vi "运维调试_采配水V3.vi"() -> ()   [LabVIEW 2016, in "PLC.lvlib"]
uses:
  PLC.lvlib
  <vilib>/Plasmionique/MB Master/MB_Master/MB_Master.lvclass
  <vilib>/Utility/miscctls.llb/LVPointTypeDef.ctl
  <vilib>/Plasmionique/MB Master/MB_Master_Serial/MB_Master_Serial.lvclass
  C:/Program Files (x86)/National Instruments/LabVIEW 2016/vi.lib/Plasmionique/MB Master/MB_Master/MB_Master.lvclass
  <vilib>/Instr/_visa.llb/VISA Configure Serial Port (Instr).vi
  <vilib>/Plasmionique/MB Master/MB Master.lvlib
panel:
  out "Registers":u16[](array[numeric])
  out "R124":i16 caption="加标回收配水时间"
  out "R44":i16
  in  "V14":bool
  in  "更新程序":bool
  out "R122":i16 caption="二级自来水清洗时间"
  out "R121":i16 caption="一级自来水清洗时间"
  out "R120":i16 caption="过滤自来水清洗时间"
  out "清洗次数":u16
  out "当前启动泵号":u16(ring) items=["1号泵", "2号泵"]
  out "R116":i16 caption="储水时间"
  in  "R113":u16(ring) caption="水箱储水水体" items=["自来水", "水样"]
  out "R112":i16 caption="二级水样池进样超时"
  in  "R111":u16(ring) caption="采配水型号" items=["常规版本", "高配版本"]
  out "数值 19":dbl
  out "数值 18":dbl
  out "数值 17":dbl
  out "数值 16":dbl
  out "数值 15":dbl
  out "数值 14":dbl
  out "数值 13":dbl
  out "数值 12":dbl
  out "数值 11":dbl
  out "数值 10":dbl
  out "数值 9":dbl
  out "数值 8":dbl
  out "数值 7":dbl
  out "数值 6":dbl
  out "数值 5":dbl
  out "数值 4":dbl
  out "数值 3":dbl
  out "数值 2":dbl
  out "数值":dbl
  in  "R118":u16(ring) caption="是否启用质控" items=["不启用质控", "启用质控"]
  out "压力传感器":dbl format="%#.2f"
  out "R110":i16 caption="过滤装置排液时间"
  in  "M4":bool
  in  "M3":bool
  in  "V13":bool
  in  "V12":bool
  in  "V1-R":bool
  in  "V1-G":bool
  in  "V11":bool
  in  "V10":bool
  in  "V9":bool
  in  "V8":bool
  in  "V7-R":bool
  in  "V7-G":bool
  out "X2":bool caption="X1"
  out "采配水版本号":string
  out "R117":i16 caption="清洗频次设定"
  out "通讯故障":bool
  in  "R100":u16(ring) caption="采水泵工作模式" items=["泵1单泵单管路", "泵2单泵单管路", "潜水泵双泵双管路", "自吸泵双泵双管路"]
  out "X11":bool caption="自来水检测_WA"
  out "X10":bool caption="废液报警_WLA"
  out "X9":bool caption="泵2过载报警_KM2"
  out "X8":bool caption="泵1过载报警_KM1"
  out "X7":bool caption="断电检测_DD"
  out "X6":bool caption="门禁开关_MJ"
  out "X5":bool caption="烟雾检测_YW"
  out "X4":bool caption="浸水检测_SJ"
  out "X3":bool caption="水流开关_JY"
  out "X1":bool
  out "X0":bool caption="采样池液位开关_YE1"
  out "R109":i16 caption="外部反冲洗时间"
  out "集成报警信息":string
  out "R108":i16 caption="进样超时时间"
  out "R107":i16 caption="进气时间"
  out "R106":i16 caption="排液时间"
  out "R105":i16 caption="常规模式配水时间"
  out "R104":i16 caption="过滤次数"
  out "R103":i16 caption="过滤配水时间"
  out "R102":i16 caption="一级沉淀时间"
  out "R101":i16 caption="管路润洗时间"
  out "R2":i16
  out "R1":i16
  out "多列列表框":i32(listbox)
  in  "V6":bool
  in  "V5":bool
  in  "V4":bool
  in  "V3":bool
  in  "V2":bool
  in  "M2":bool
  in  "M1":bool
  in  "返回":bool
  in  "参数设置":bool
  in  "单步启动":bool
  in  "启动":bool
  in  "停止":bool
  # "流程计时："
  # "s"
  # "压力传感器："
  # "MPa"
  # "二级液位开关低_Y2FD"
  # "二级液位开关高_YF2H"
  # "S"
  # "S"
  # "S"
  # "S"
  # "S"
  # "S"
  # "次"
  # "S"
  # "S"
  # "S"
  # "S"
  # "S"
  # "S"
  # "单步计时："
  # "s"
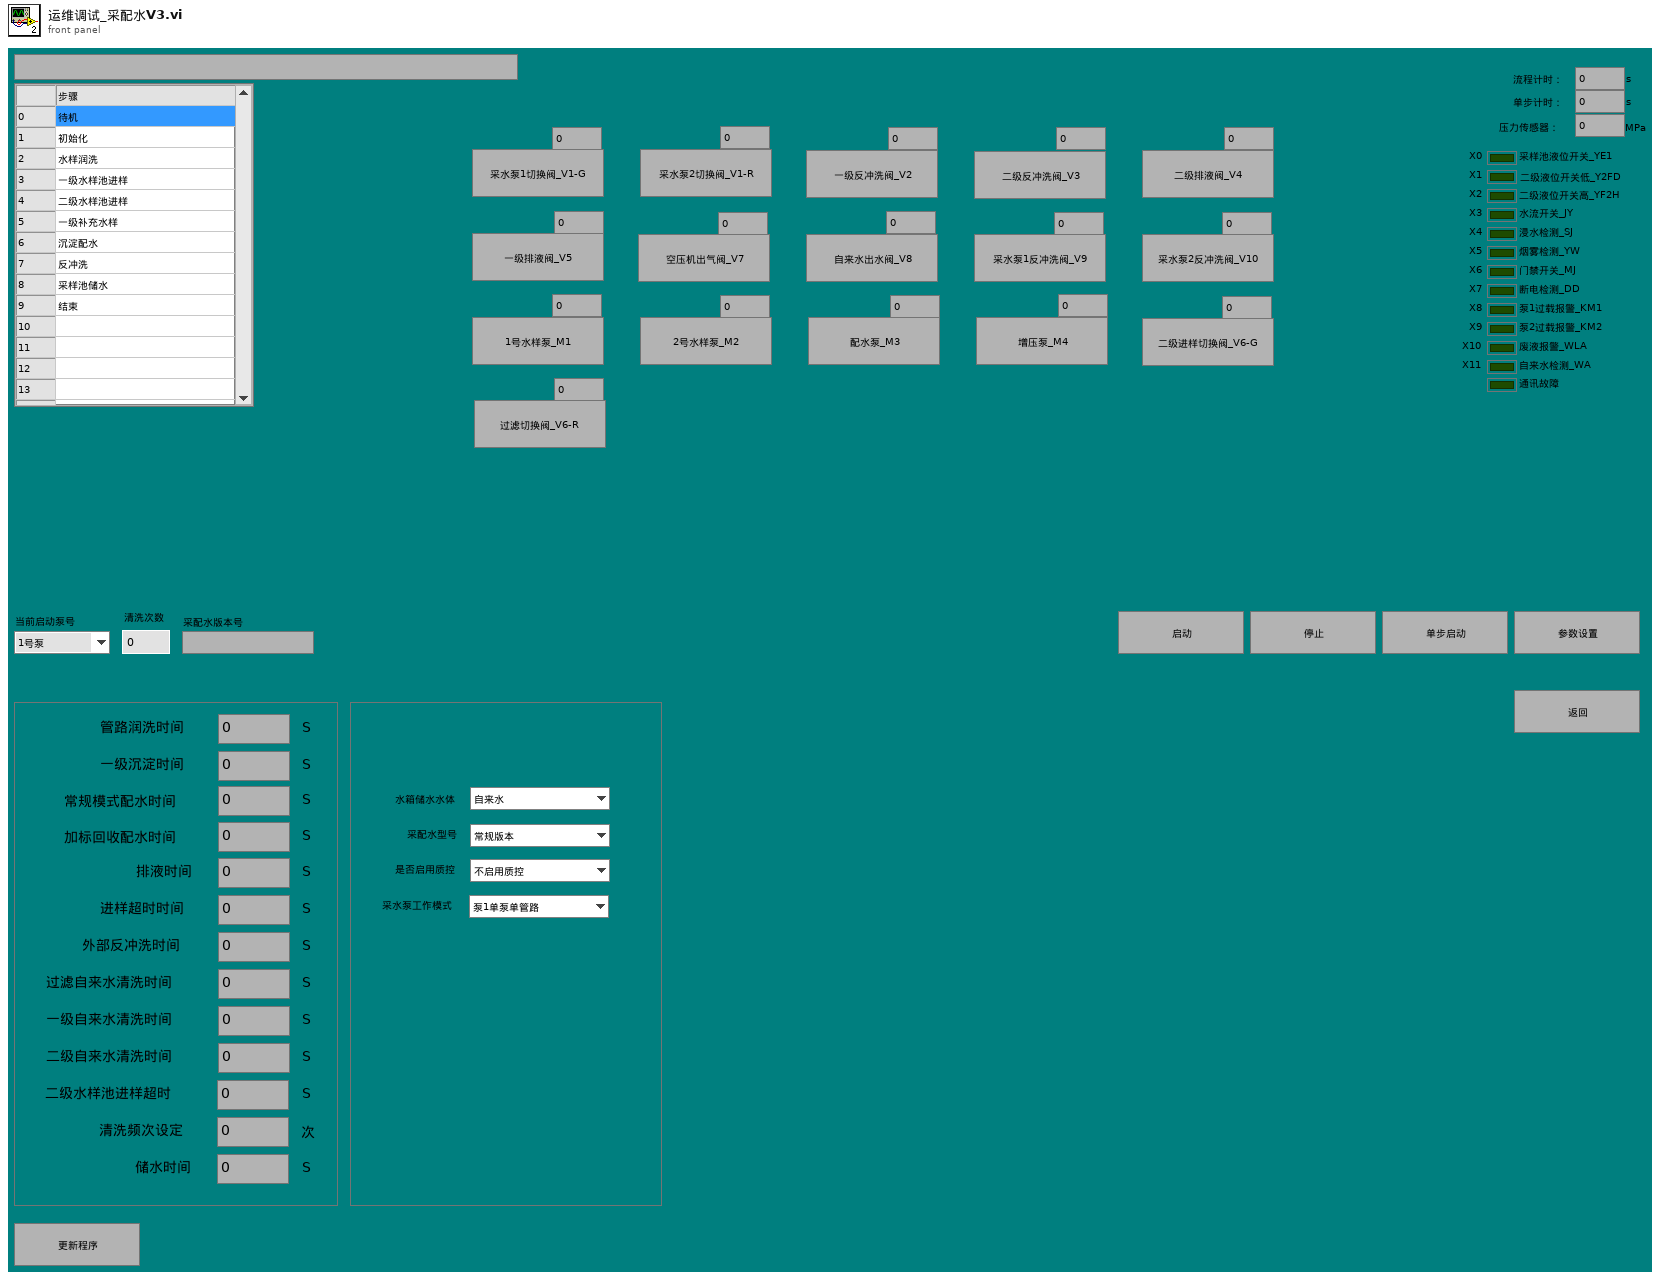
[diagram p1: front panel]
types:
  T1 = cluster{"测试模式":enum16{"水样测试", "平行样测试", "集成干预测试", "加标回收"}, "参数启用":cluster{"氨氮":bool, "总磷":bool, "总氮":bool, "多参数":bool, "CODMn":bool, "CODcr":bool, "超标留样":bool}}
  T2 = typedef "LVPointTypeDef.ctl" = cluster{"Horizontal":i16, "Vertical":i16}
  T3 = cluster{"命令":string, "数据":cluster{"starting address":u16, "holding register value":u16}}
  T4 = cluster{"命令":string, cluster{"starting address":u16, "holding register value":u16}}
  T5 = cluster{"命令":string, "数据":cluster{"starting address":u16, "holding register values":u16[]}}
  T6 = cluster{"命令":string, "data":cluster{"starting address":u16, "coil values":bool[]}}
  T7 = cluster{"参数启用":cluster{"氨氮":bool, "总磷总氮":bool, "总氮":bool, "多参数":bool, "CODMn":bool, "CODcr":bool, "超标留样":bool}}
  T8 = cluster{"氨氮":bool, "总磷总氮":bool, "总氮":bool, "多参数":bool, "CODMn":bool, "CODcr":bool, "超标留样":bool}
  T9 = cluster{"测试模式":enum16{"水样测试", "平行样测试", "集成干预测试", "加标回收"}, "参数启用":cluster{"氨氮":bool, "总磷总氮":bool, "总氮":bool, "多参数":bool, "CODMn":bool, "CODcr":bool, "超标留样":bool}}
  T10 = cluster{"R0":i16, "R1":i16, "R2":i16, "R3":i16, "R4":i16, "R5":i16, "R6":i16, "R7":i16, "R8":i16, "R9":i16, "R10":i16, "R11":i16, "R12":i16, "R13":i16, "R14":i16, "R15":i16, "R16":i16, "R17":i16, "R18":i16, "R19":i16, "R20":i16, "R21":i16, "R22":i16, "R23":i16, "R24":i16, "R25":i16, "R26":i16, "R27":i16, "R28":i16, "R29":i16, "R30":i16, "R31":i16, "R32":i16, "R33":i16, "R34":i16, "R35":i16, "R36":i16, "R37":i16, "R38":i16, "R39":i16, "R40":i16, "R41":i16, "R42":i16, "R43":i16, "R44":i16, "R45":i16, "R46":i16, "R47":i16, "R48":i16, "R49":i16, "R50":i16, "R51":i16, "R52":i16, "R53":i16, "R54":i16, "R55":i16, "R56":i16, "R57":i16, "R58":i16, "R59":i16, "R60":i16, "R61":i16, "R62":i16, "R63":i16, "R64":i16, "R65":i16, "R66":i16, "R67":i16, "R68":i16, "R69":i16, "R70":i16, "R71":i16, "R72":i16, "R73":i16, "R74":i16, "R75":i16, "R76":i16, "R77":i16, "R78":i16, "R79":i16}
  T11 = cluster{"seconds since 1Jan1904":timestamp, "table输入":string, string, "table输入":string}
  T12 = cluster{"baud rate (bps)":u32, "stop bits":u16, "parity":u16, "flow control":u16, "timeout":u32, "retries":i32}
  T13 = cluster{"starting address":u16, "holding register values":u16[]}
  T14 = cluster{"starting address":u16, "holding register value":u16}
  T15 = cluster{"starting address":u16, "coil values":bool[]}
  T16 = cluster{"Registers[0]":u16, "Registers[1]":u16, "Registers[2]":u16, "Registers[3]":u16, "Registers[4]":u16, "Registers[5]":u16, "Registers[6]":u16, "Registers[7]":u16, "Registers[8]":u16, "Registers[9]":u16, "Registers[10]":u16, "Registers[11]":u16, "Registers[12]":u16, "Registers[13]":u16, "Registers[14]":u16, "Registers[15]":u16, "Registers[16]":u16, "Registers[17]":u16, "Registers[18]":u16, "Registers[19]":u16, "Registers[20]":u16, "Registers[21]":u16, "Registers[22]":u16, "Registers[23]":u16, "Registers[24]":u16, "Registers[25]":u16, "Registers[26]":u16, "Registers[27]":u16, "Registers[28]":u16, "Registers[29]":u16, "Registers[30]":u16, "Registers[31]":u16, "Registers[32]":u16, "Registers[33]":u16, "Registers[34]":u16, "Registers[35]":u16, "Registers[36]":u16, "Registers[37]":u16, "Registers[38]":u16, "Registers[39]":u16, "Registers[40]":u16, "Registers[41]":u16, "Registers[42]":u16, "Registers[43]":u16, "Registers[44]":u16, "Registers[45]":u16, "Registers[46]":u16, "Registers[47]":u16, "Registers[48]":u16, "Registers[49]":u16, "Registers[50]":u16, "Registers[51]":u16, "Registers[52]":u16, "Registers[53]":u16, "Registers[54]":u16, "Registers[55]":u16, "Registers[56]":u16, "Registers[57]":u16, "Registers[58]":u16, "Registers[59]":u16, "Registers[60]":u16, "Registers[61]":u16, "Registers[62]":u16, "Registers[63]":u16, "Registers[64]":u16, "Registers[65]":u16, "Registers[66]":u16, "Registers[67]":u16, "Registers[68]":u16, "Registers[69]":u16, "Registers[70]":u16, "Registers[71]":u16, "Registers[72]":u16, "Registers[73]":u16, "Registers[74]":u16, "Registers[75]":u16, "Registers[76]":u16, "Registers[77]":u16, "Registers[78]":u16, "Registers[79]":u16}
  T17 = cluster{"Registers[0]":u16, "Registers[1]":u16, "Registers[2]":u16, "Registers[3]":u16, "Registers[4]":u16, "Registers[5]":u16}
  T18 = cluster{"Registers[0]":u16, "Registers[1]":u16, "Registers[2]":u16, "Registers[3]":u16, "Registers[4]":u16, "Registers[5]":u16, "Registers[6]":u16, "Registers[7]":u16, "Registers[8]":u16, "Registers[9]":u16, "Registers[10]":u16, "Registers[11]":u16, "Registers[12]":u16, "Registers[13]":u16, "Registers[14]":u16, "Registers[15]":u16, "Registers[16]":u16, "Registers[17]":u16, "Registers[18]":u16, "Registers[19]":u16, "Registers[20]":u16, "Registers[21]":u16, "Registers[22]":u16, "Registers[23]":u16, "Registers[24]":u16, "Registers[25]":u16, "Registers[26]":u16, "Registers[27]":u16, "Registers[28]":u16, "Registers[29]":u16, "Registers[30]":u16, "Registers[31]":u16, "Registers[32]":u16, "Registers[33]":u16}
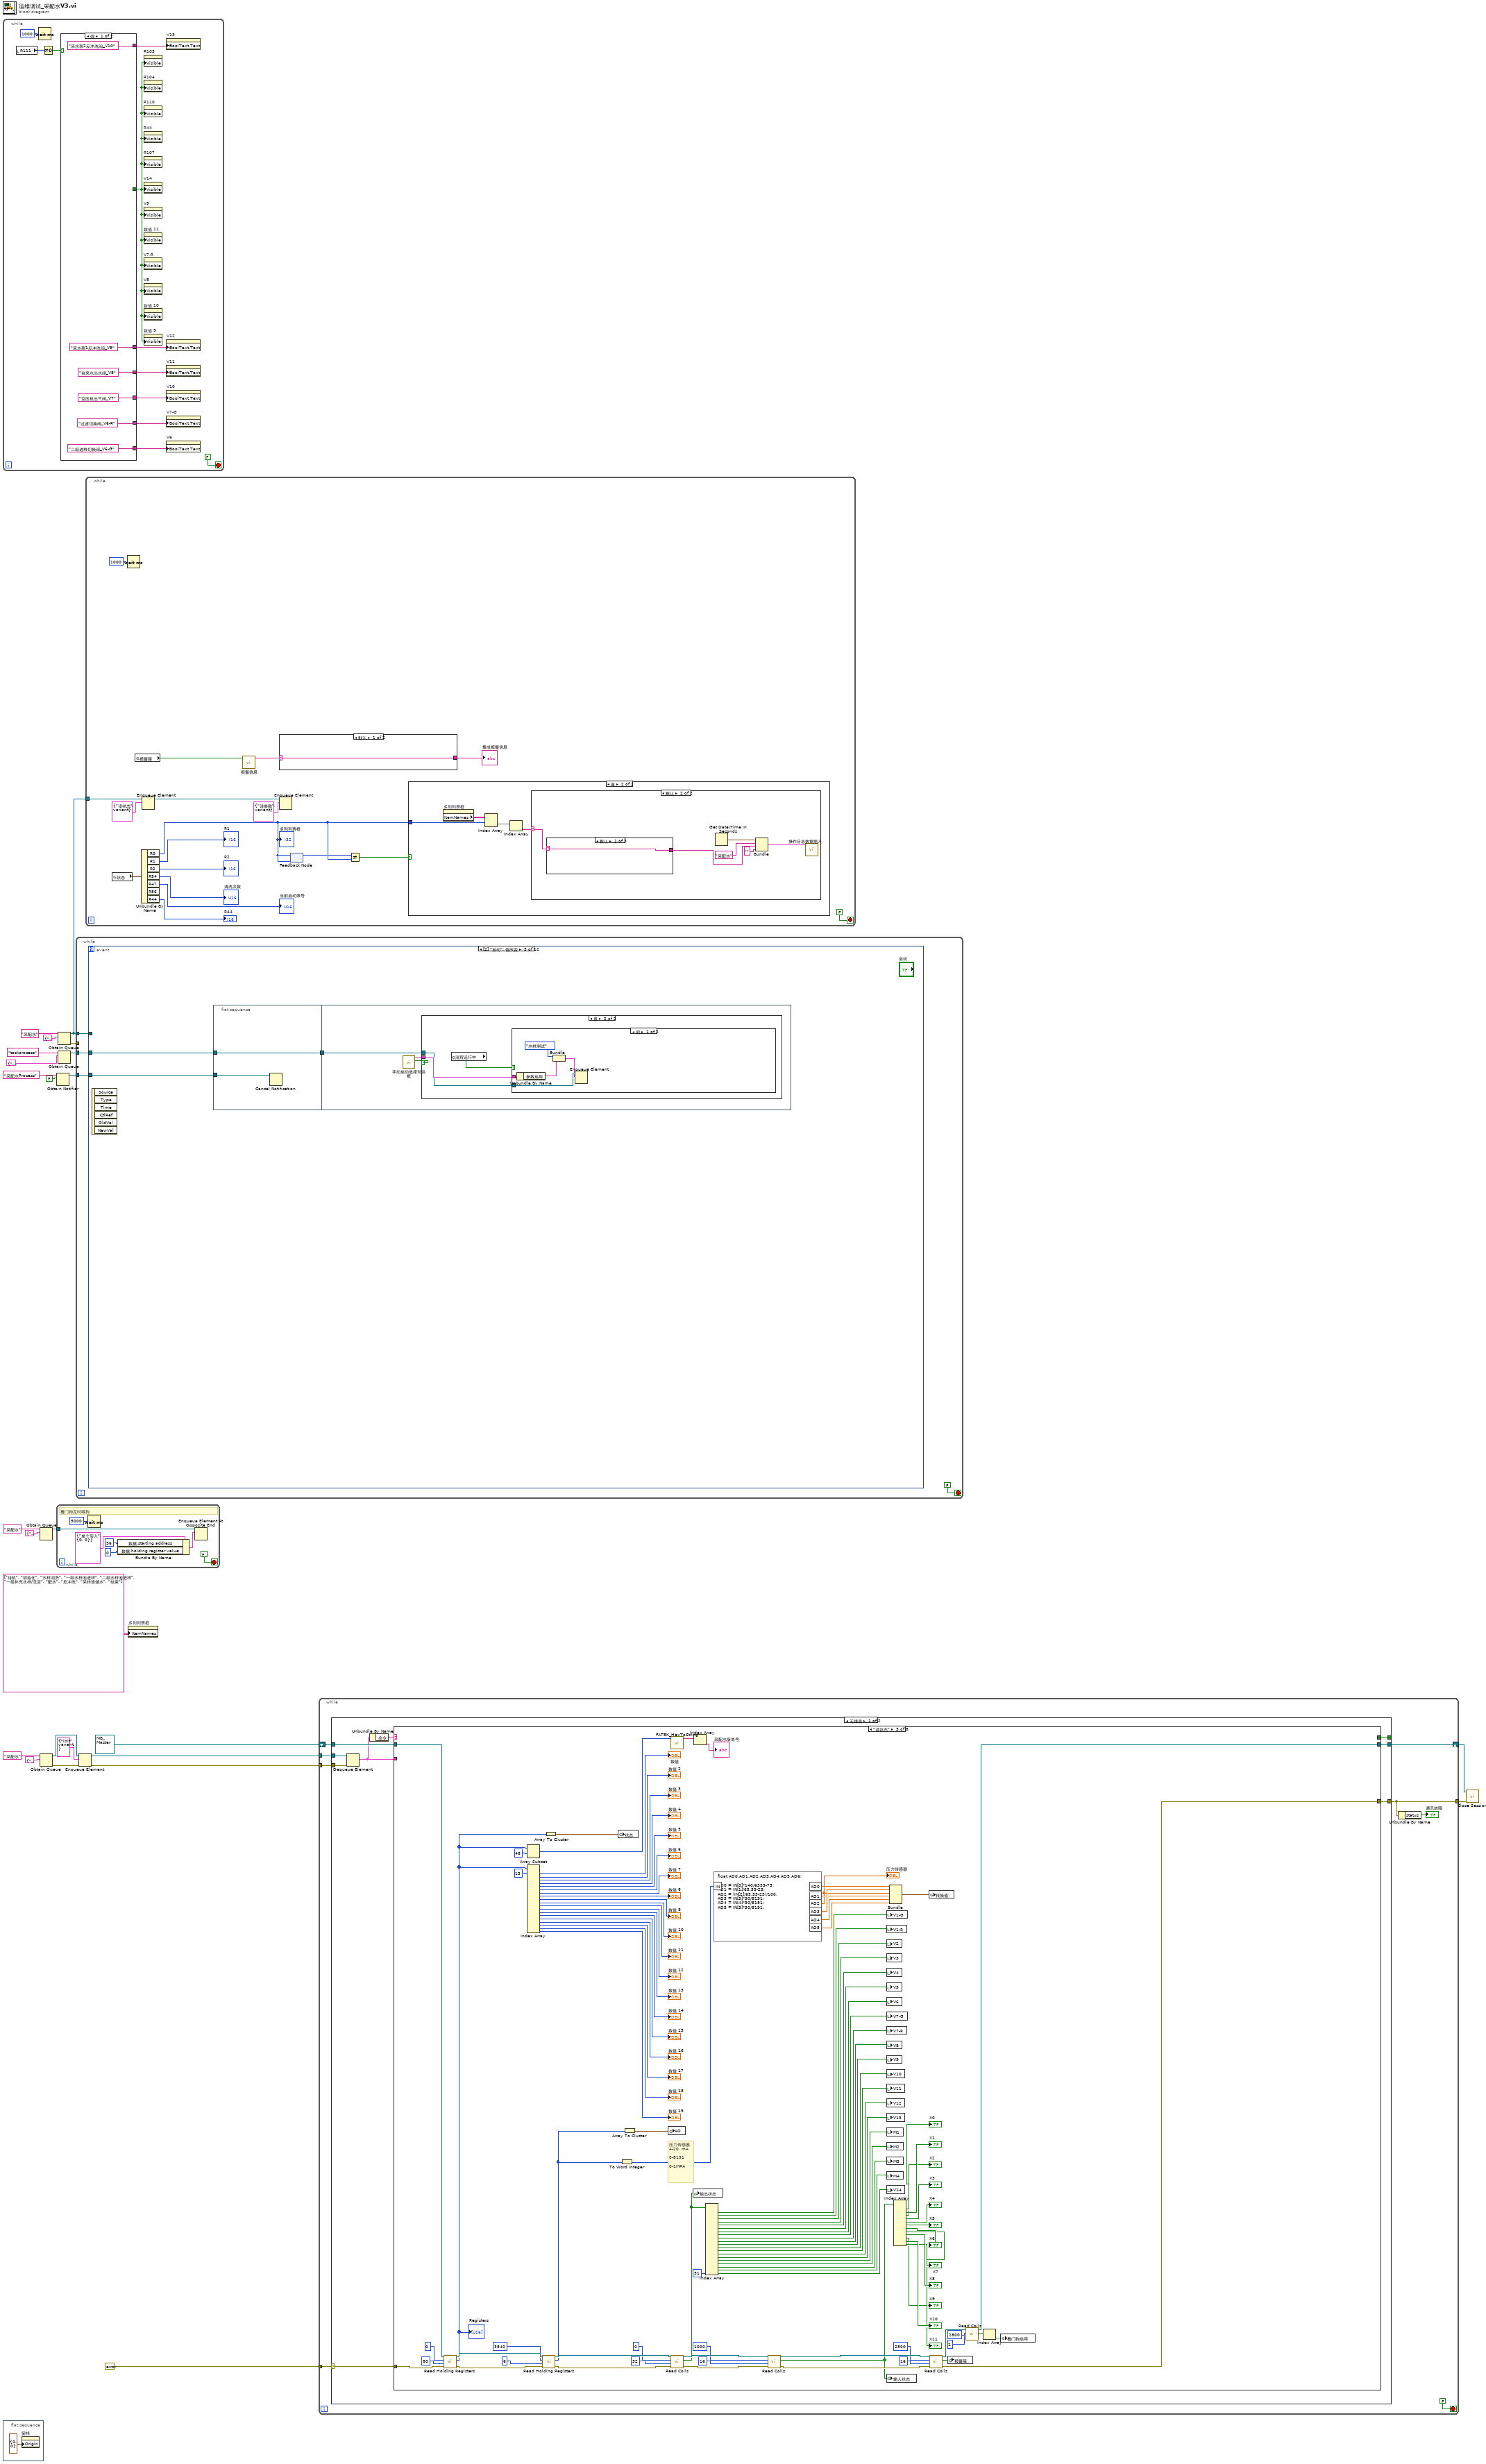
[diagram p0: block diagram]
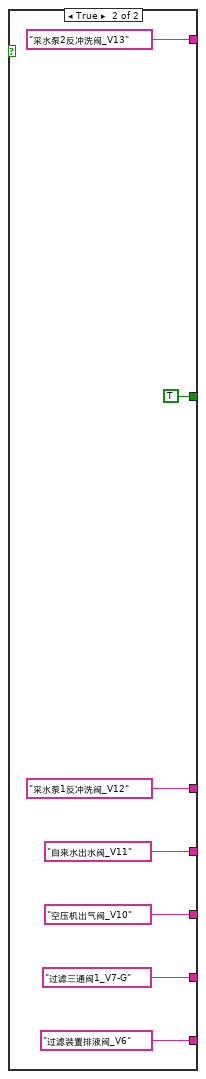
[diagram p2: hidden frame]
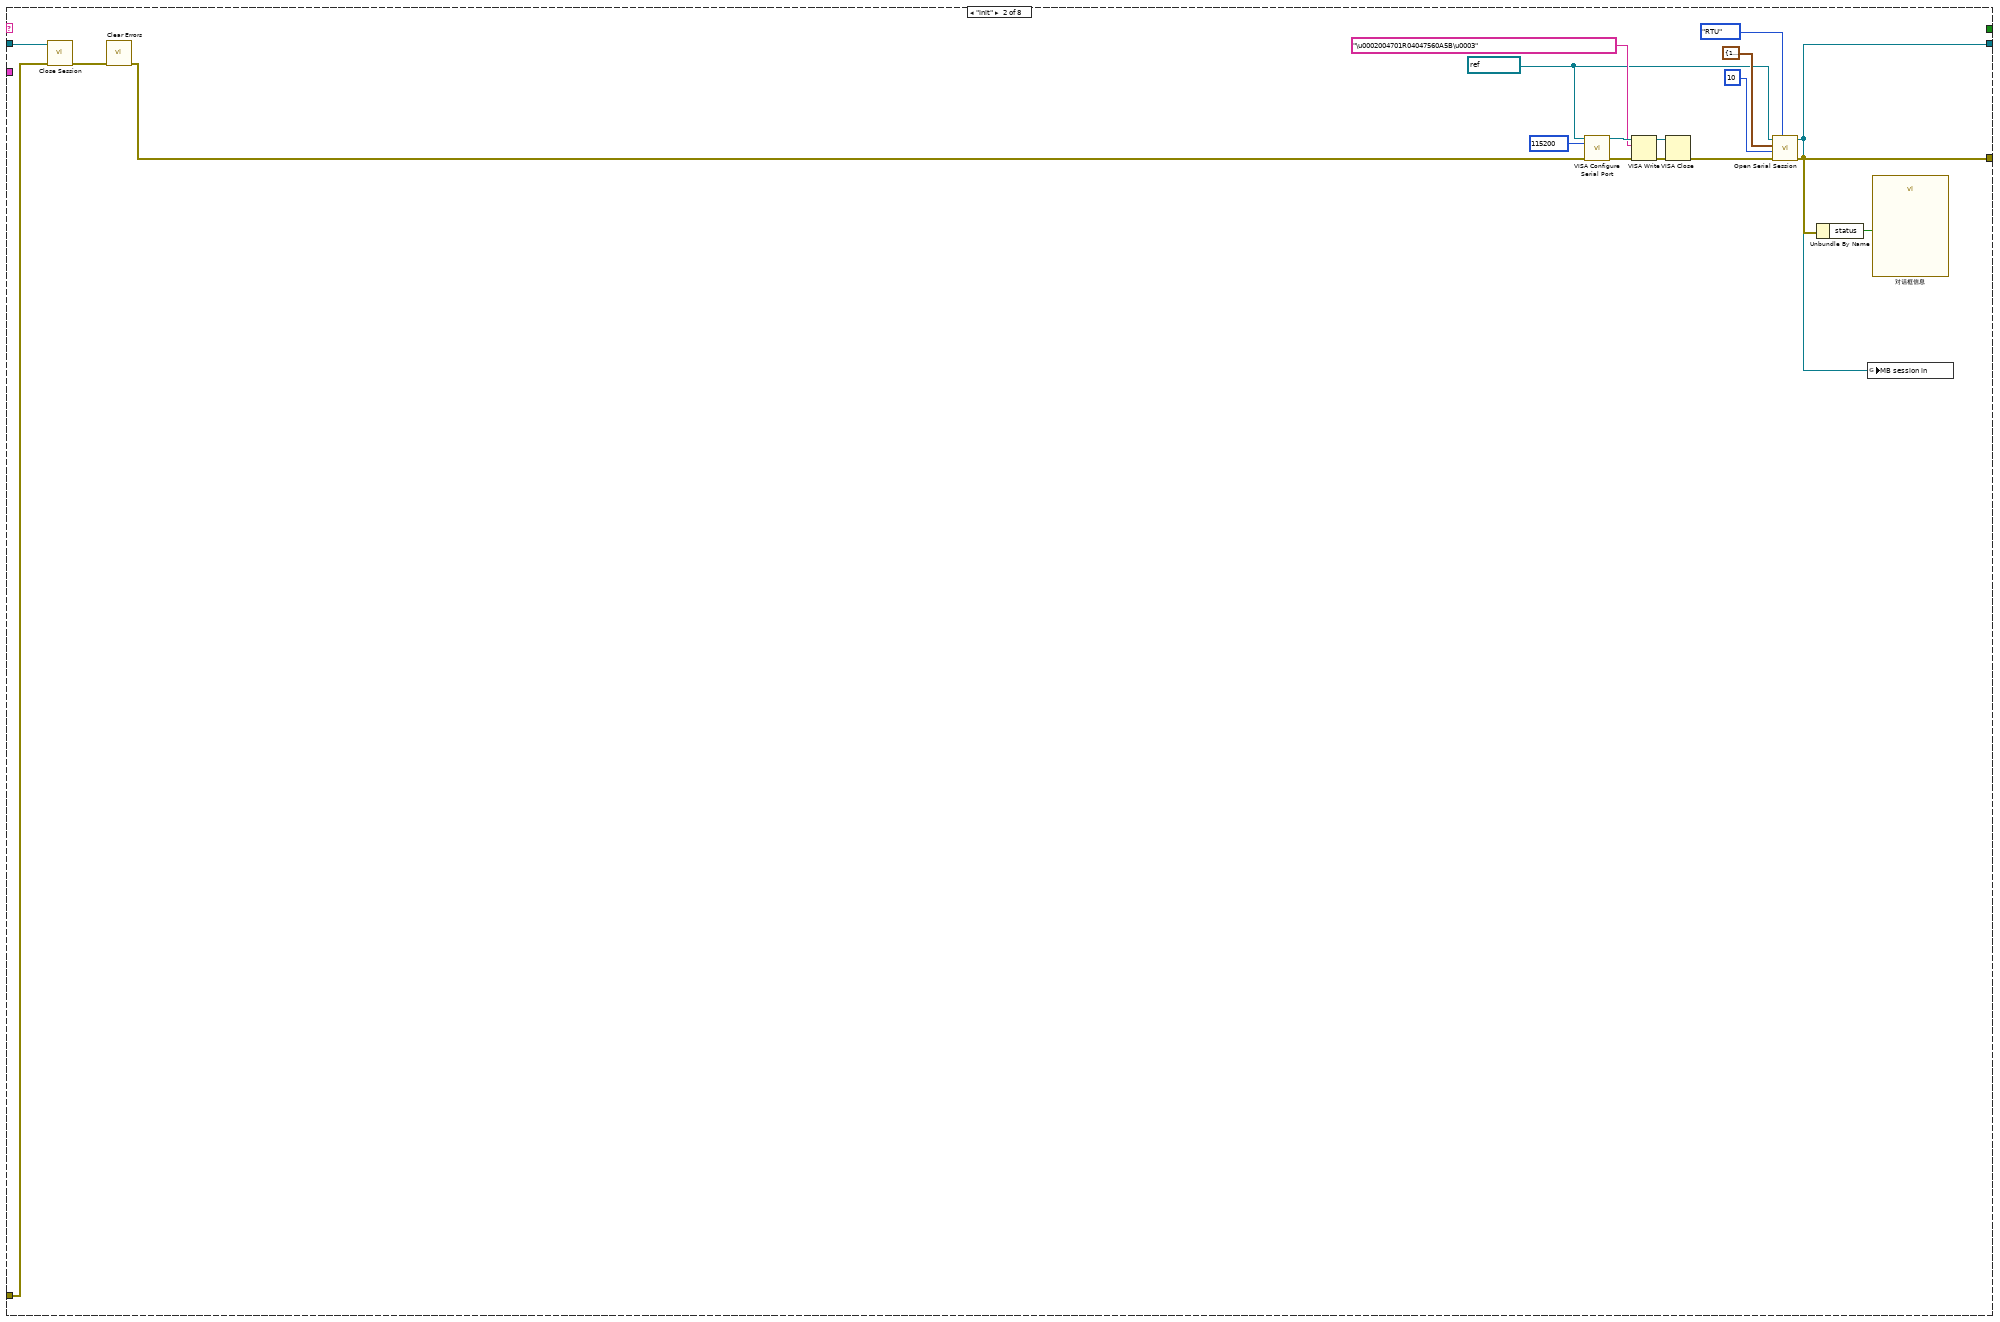
[diagram p4: hidden frame]
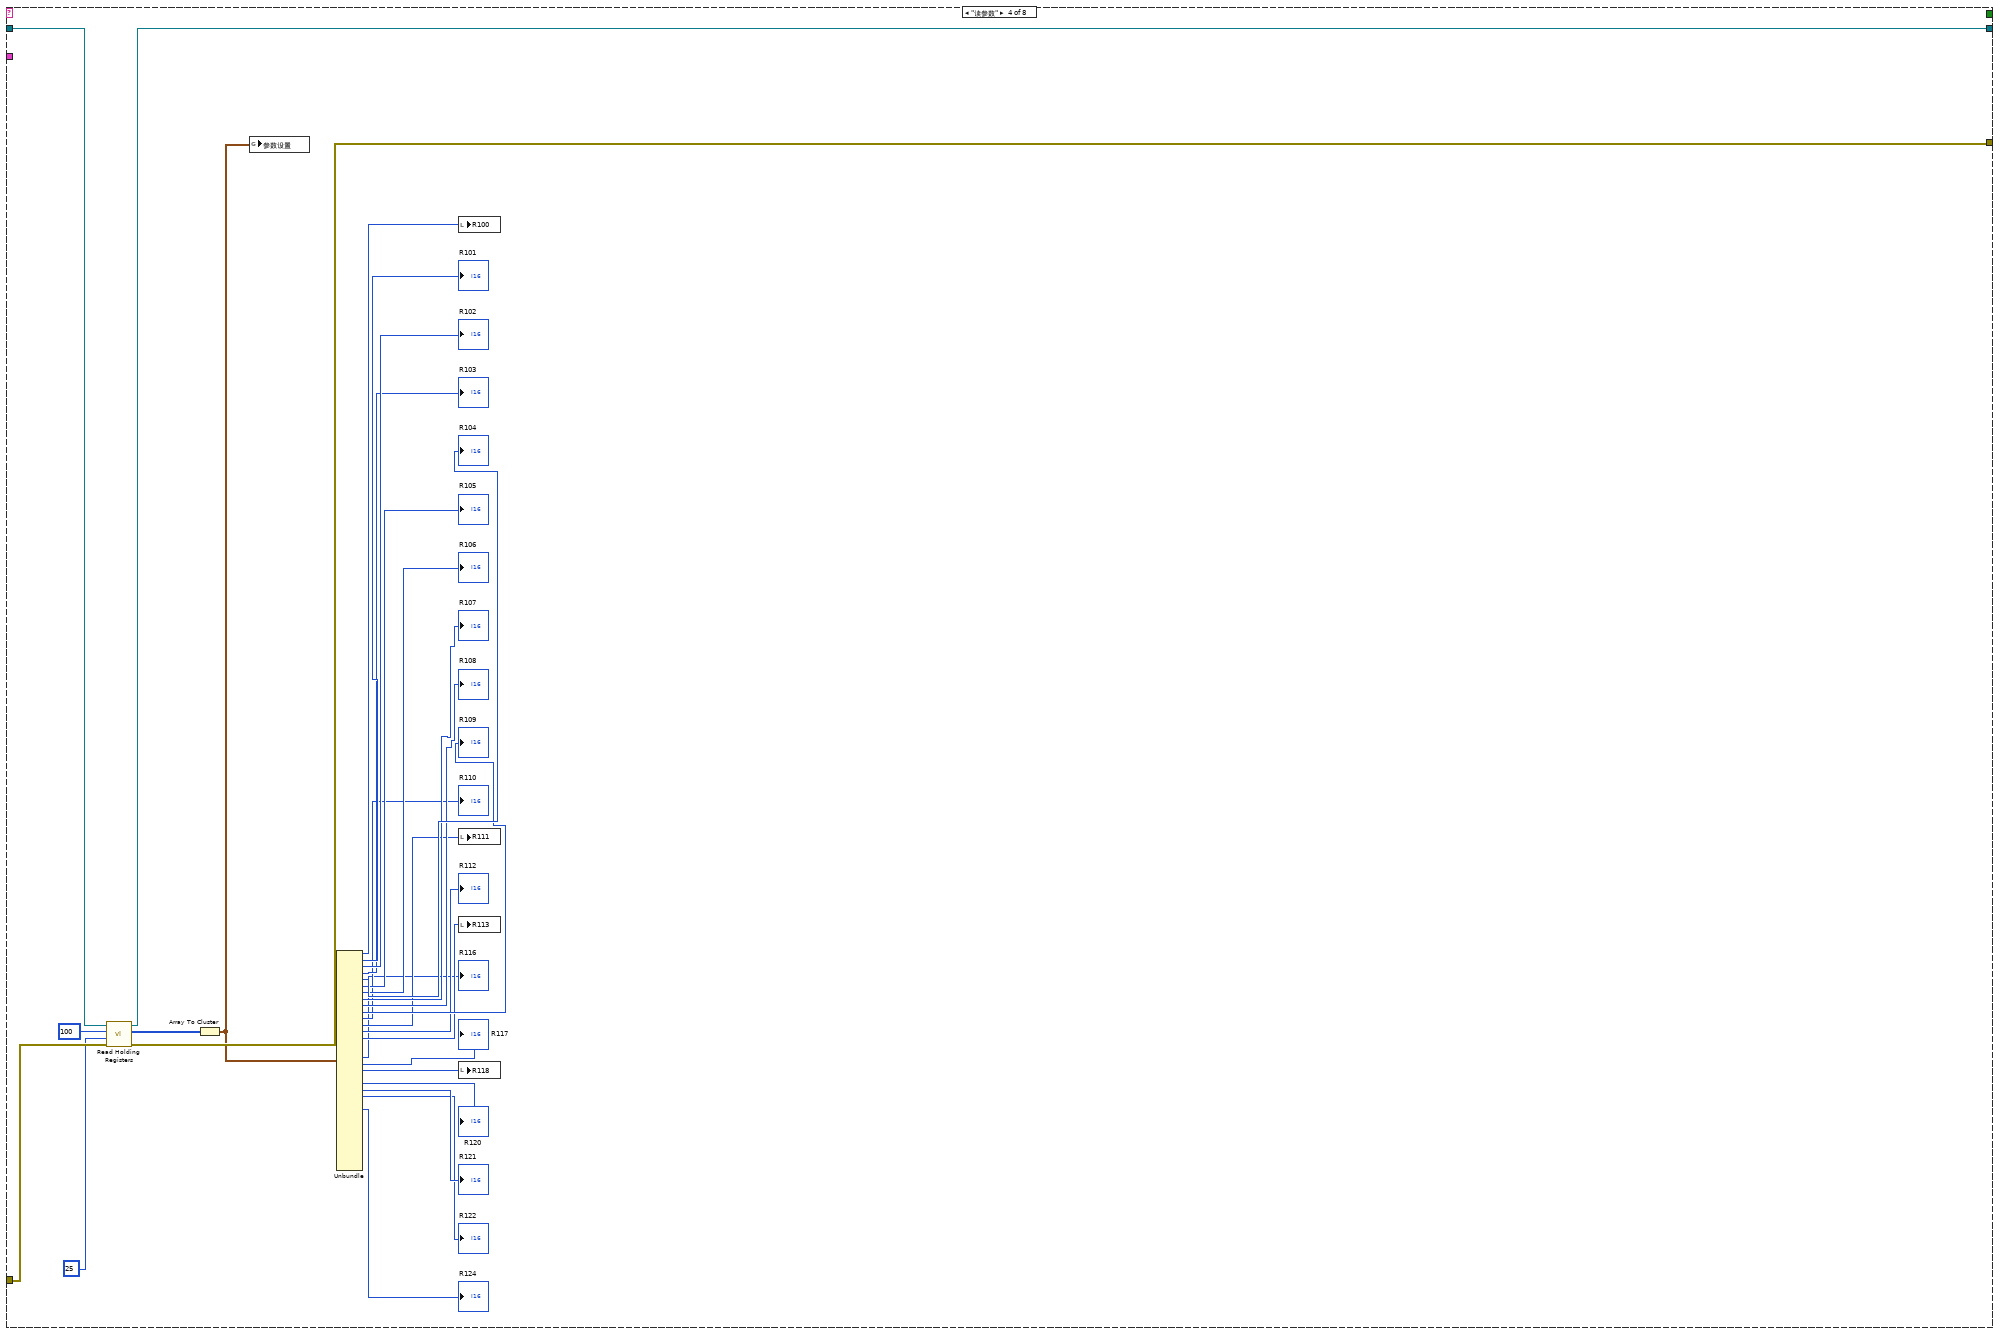
[diagram p5: hidden frame]
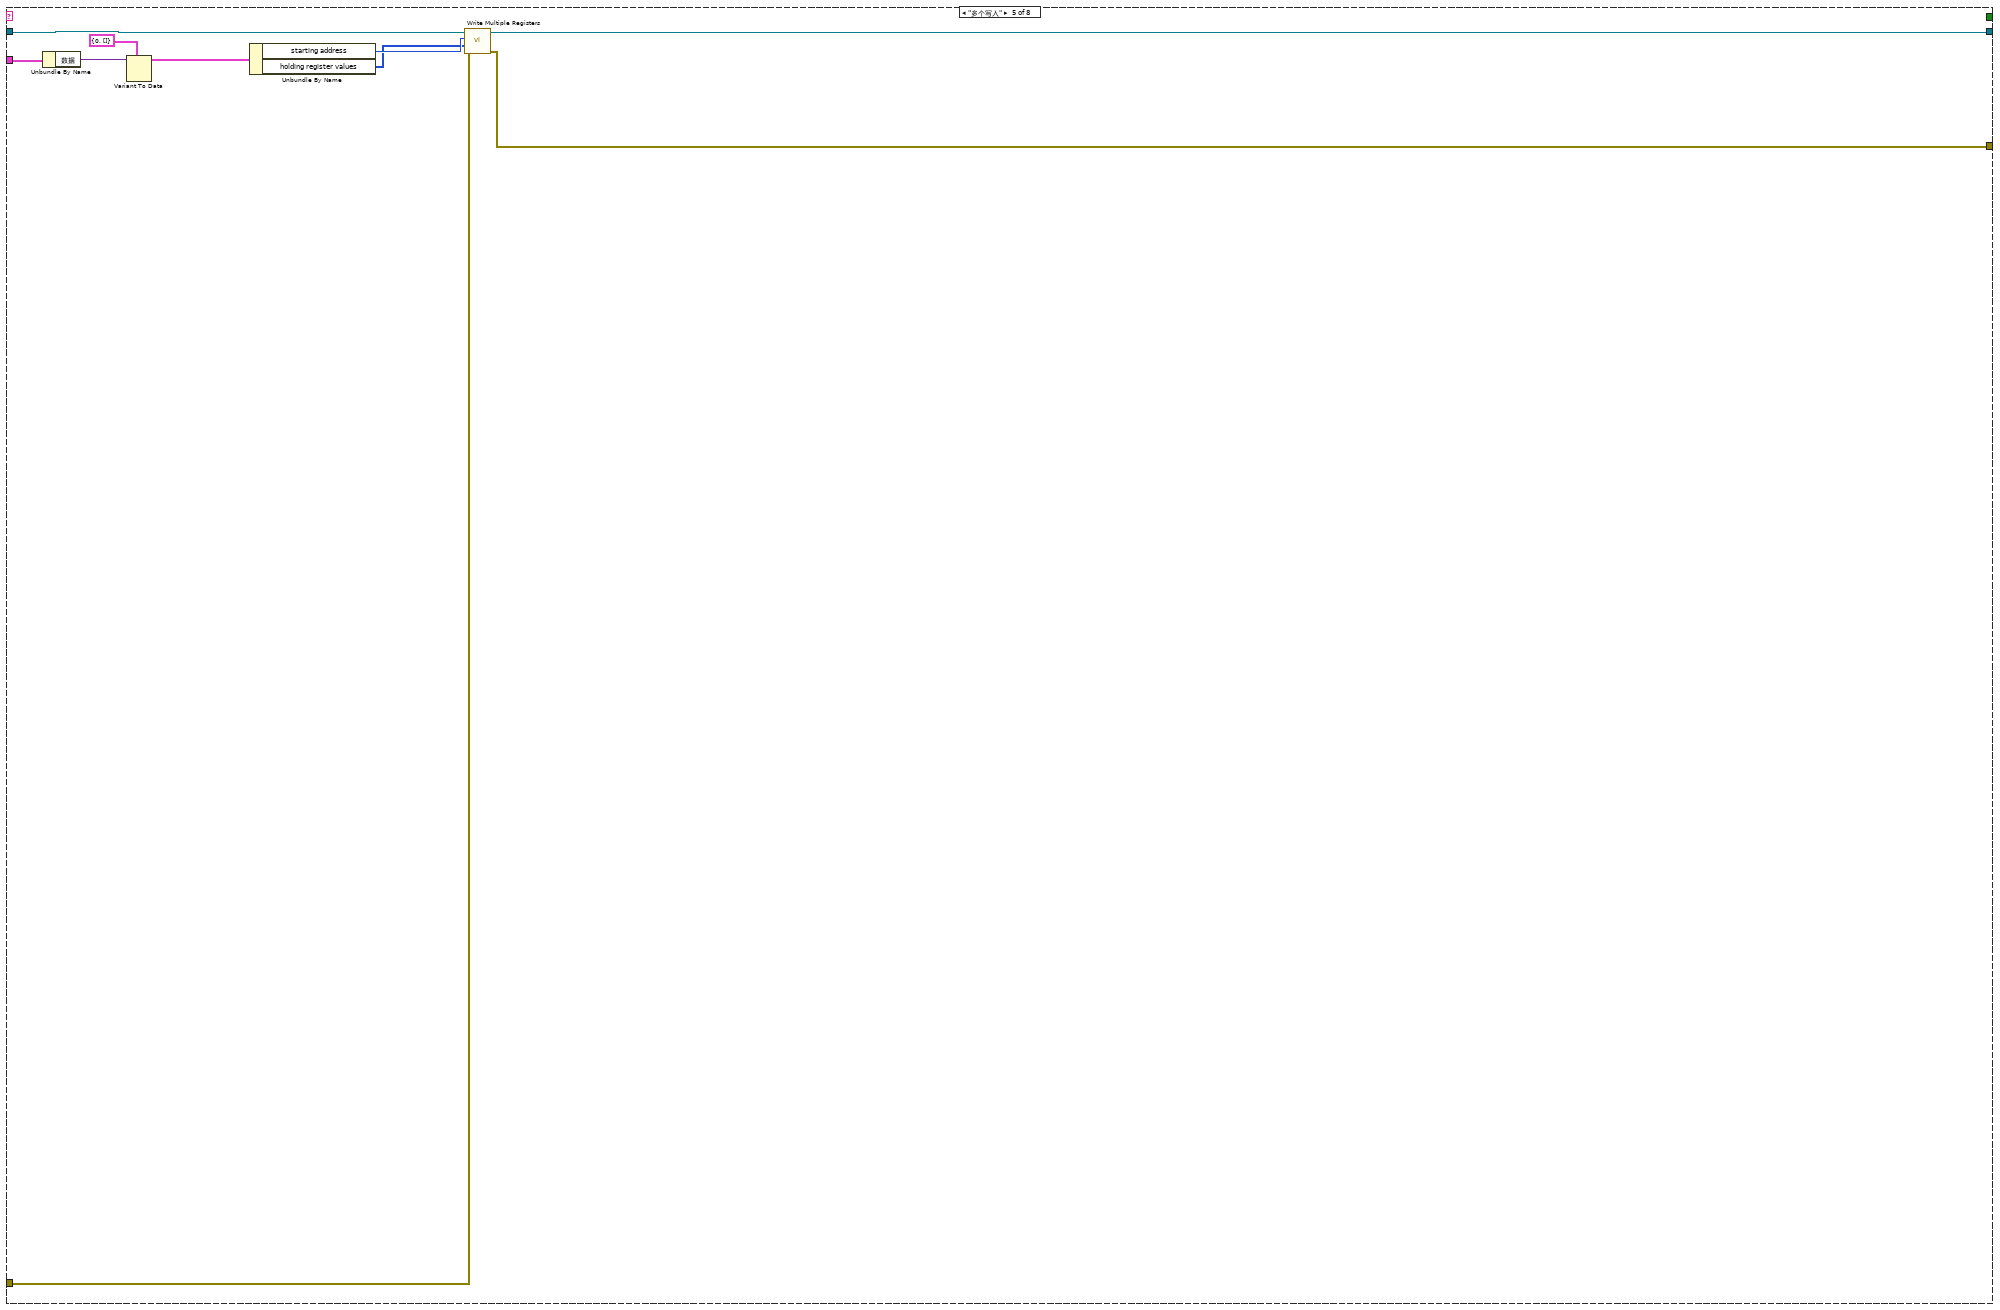
[diagram p6: hidden frame]
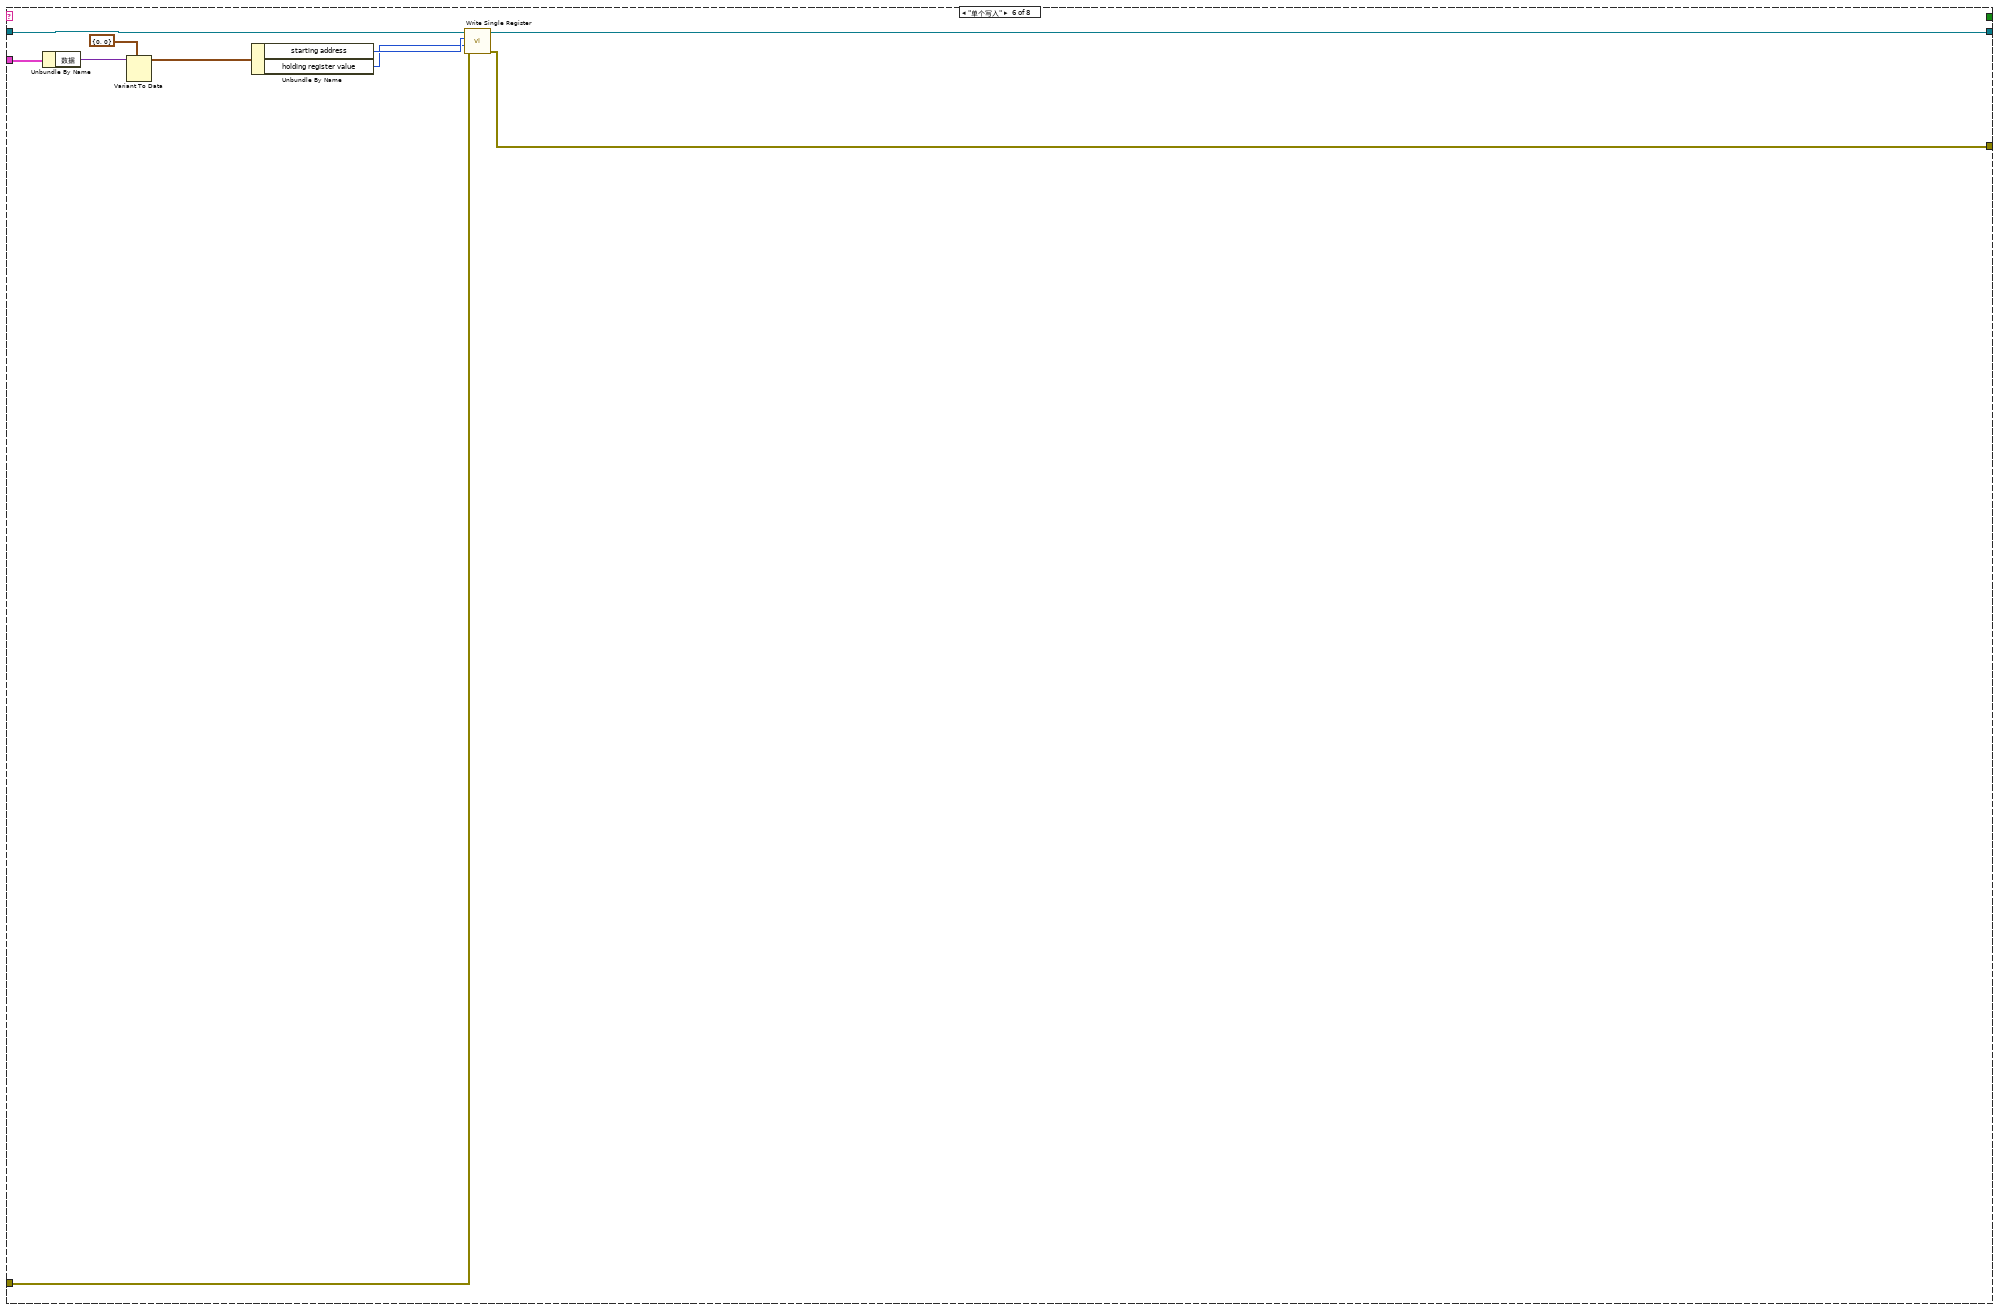
[diagram p7: hidden frame]
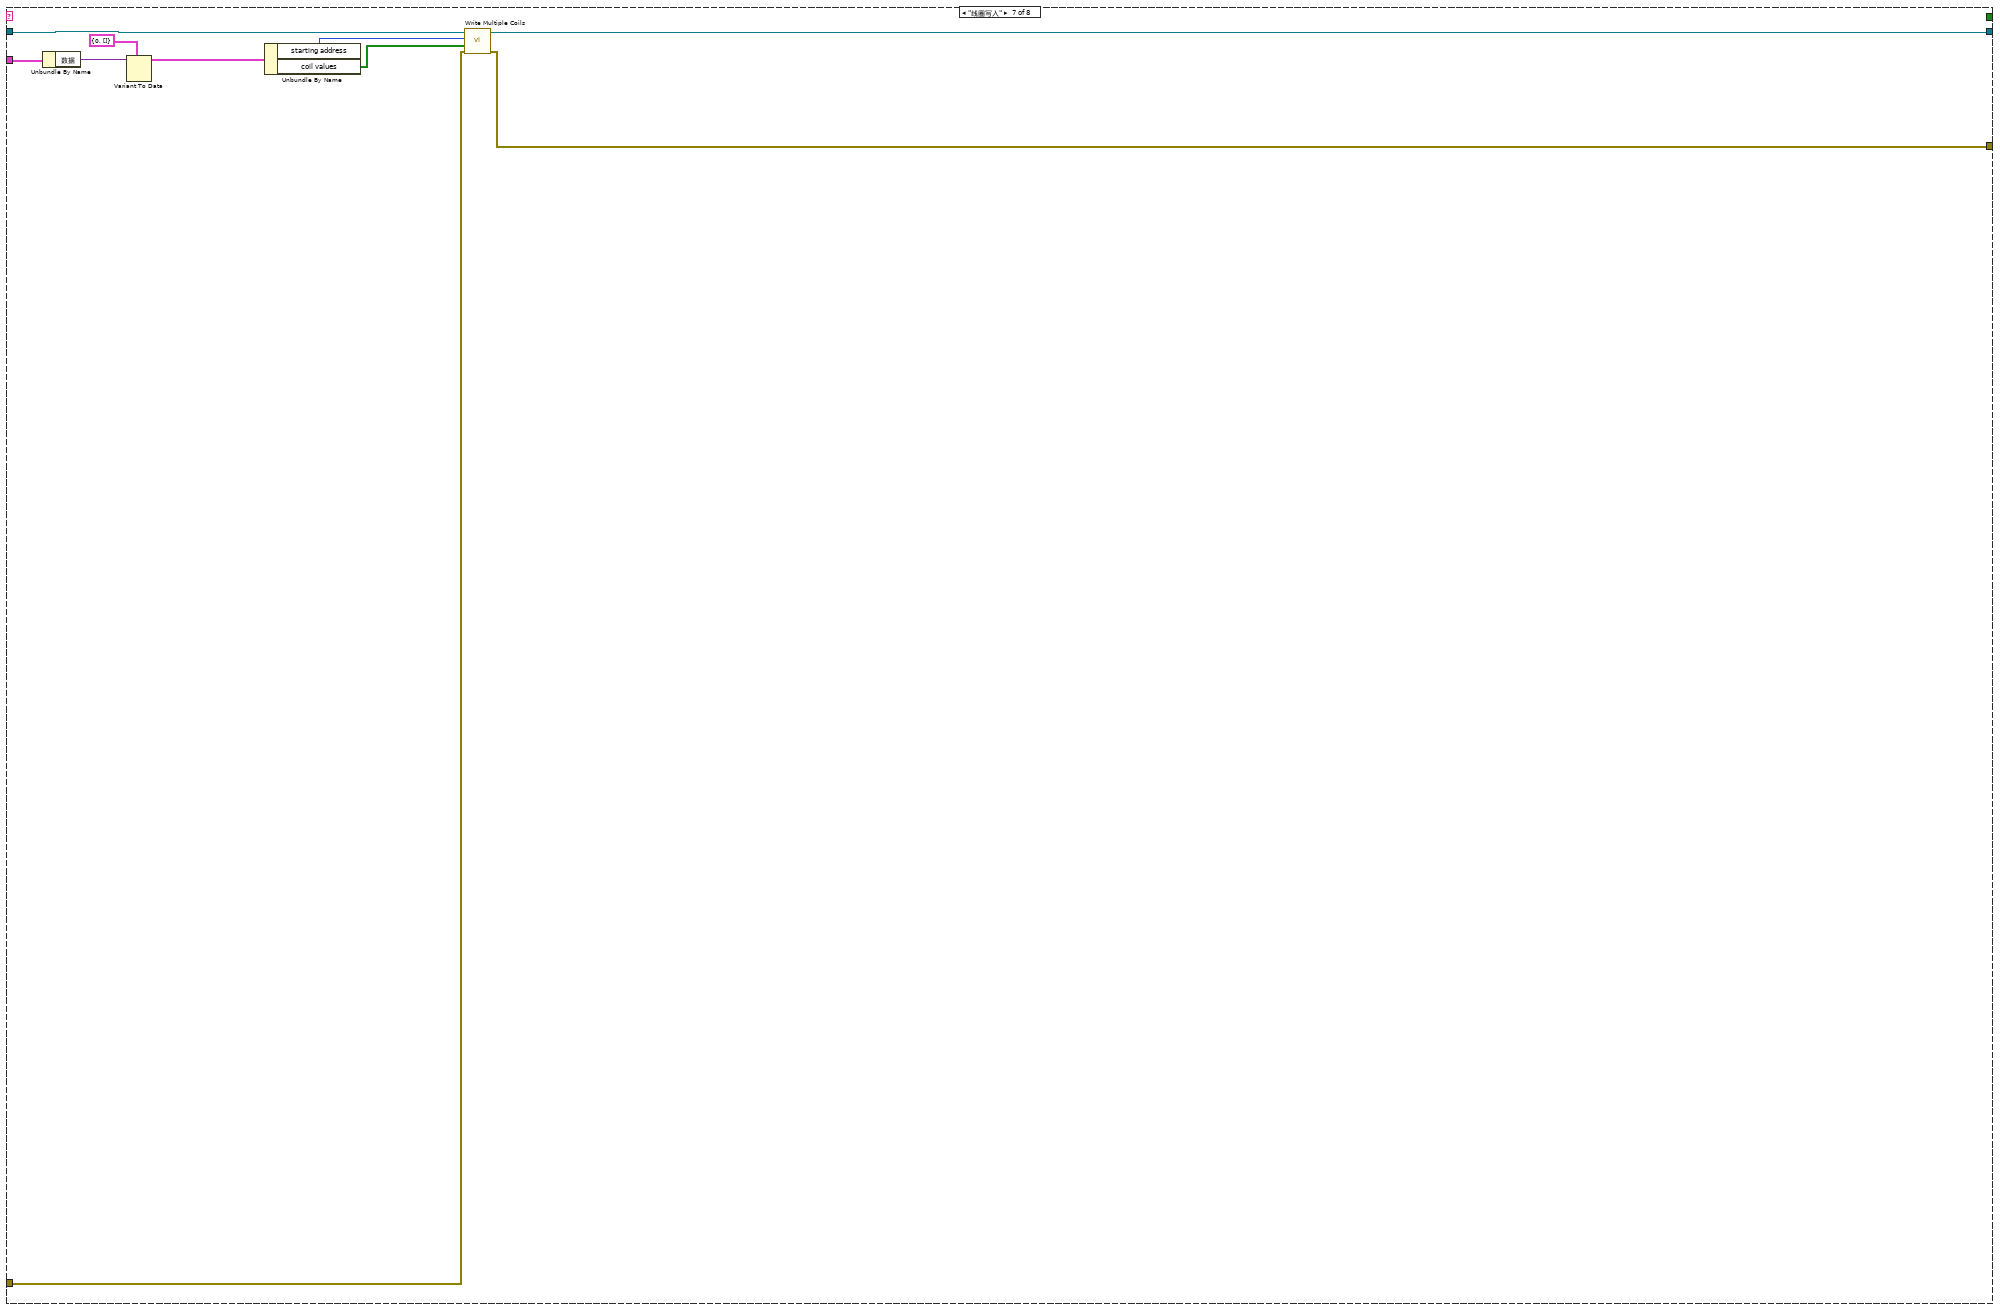
[diagram p8: hidden frame]
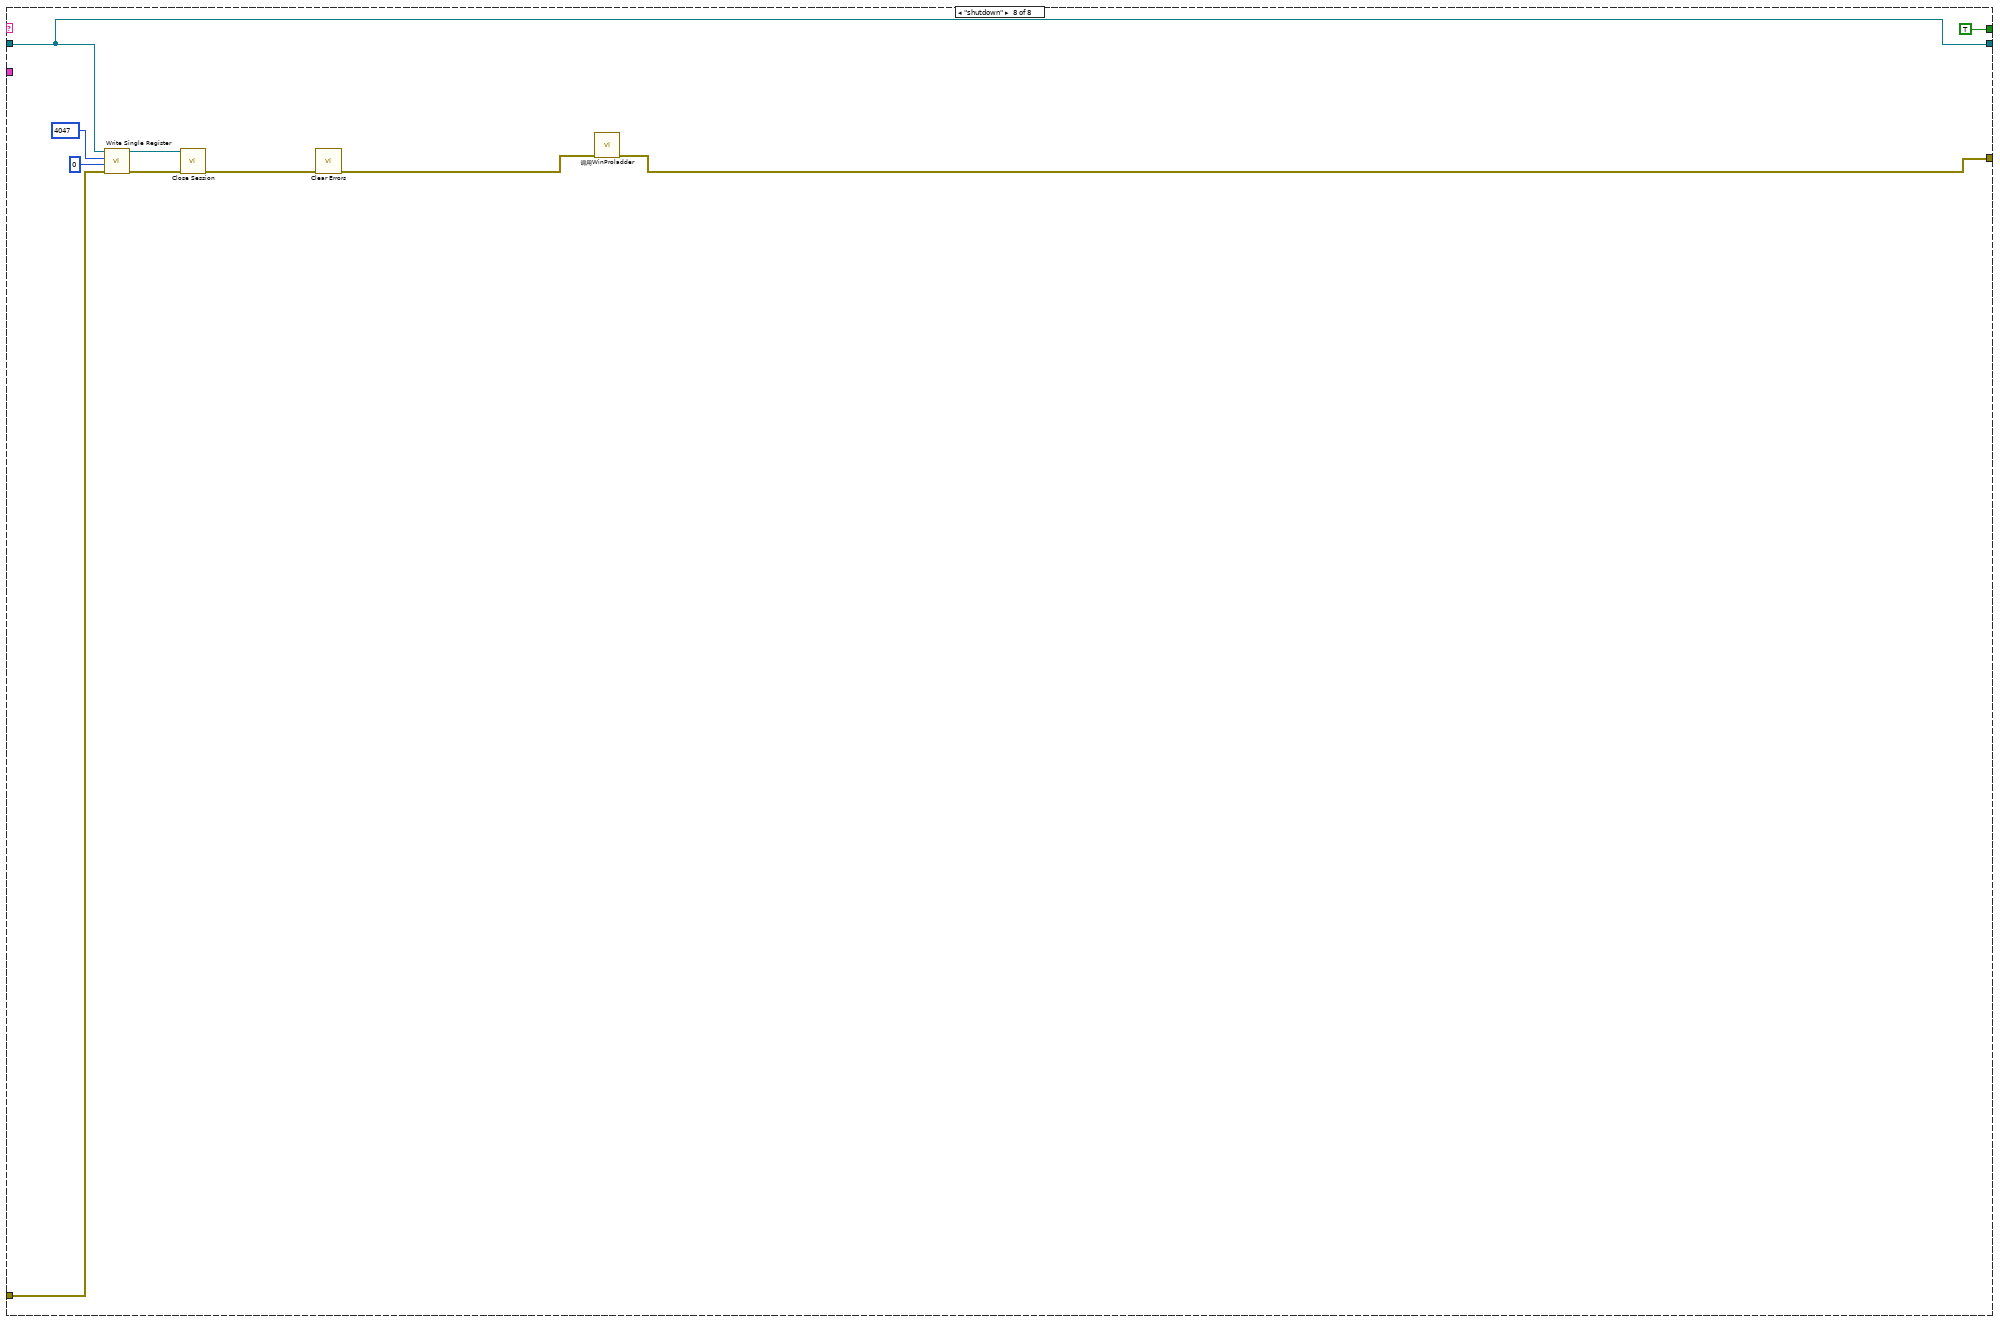
[diagram p9: hidden frame]
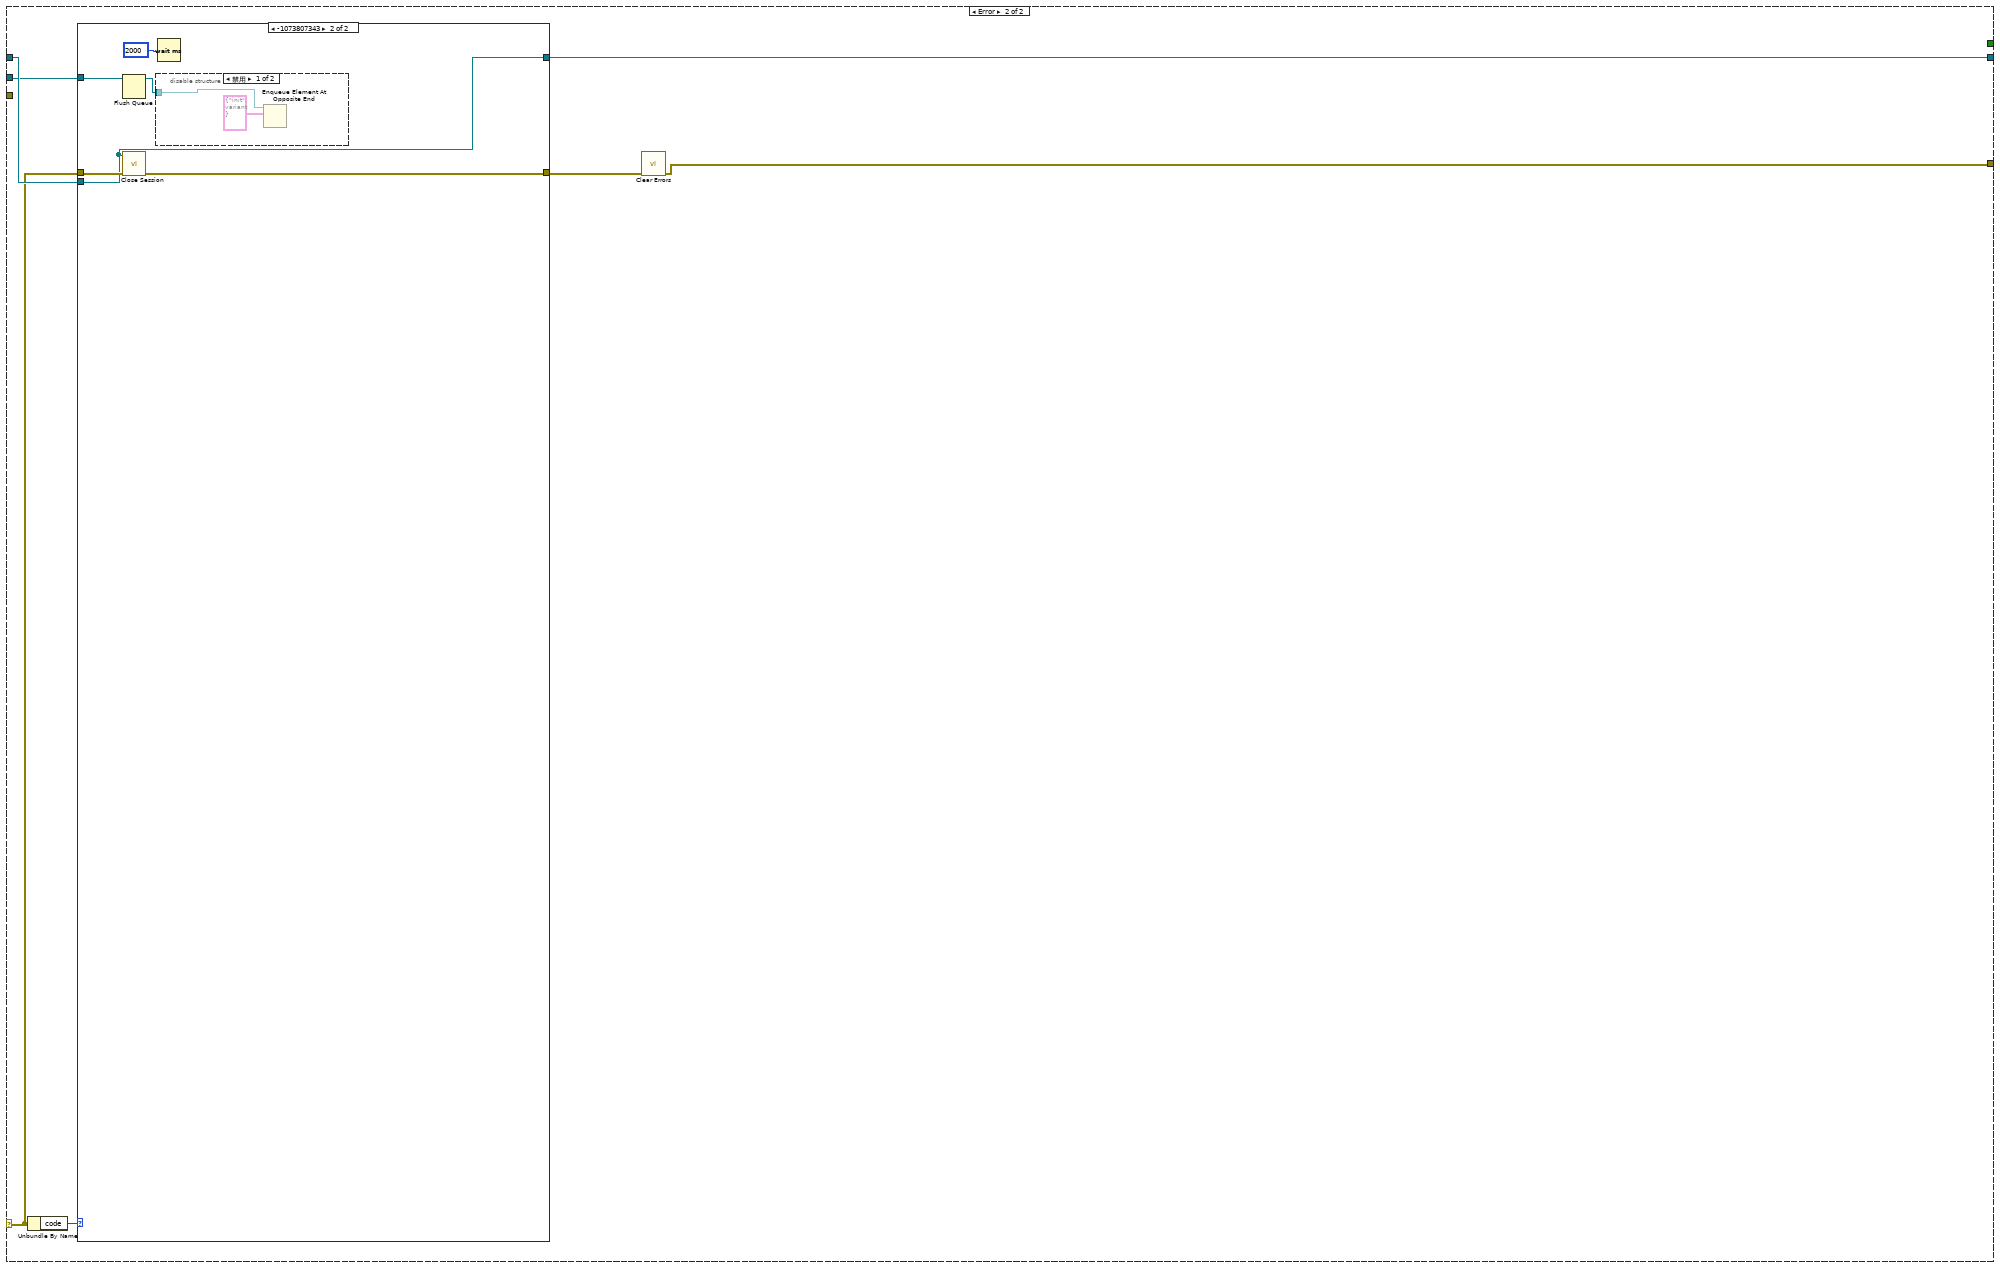
[diagram p10: hidden frame]
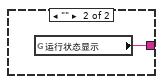
[diagram p13: hidden frame]
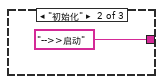
[diagram p16: hidden frame]
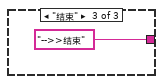
[diagram p17: hidden frame]
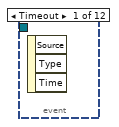
[diagram p18: hidden frame]
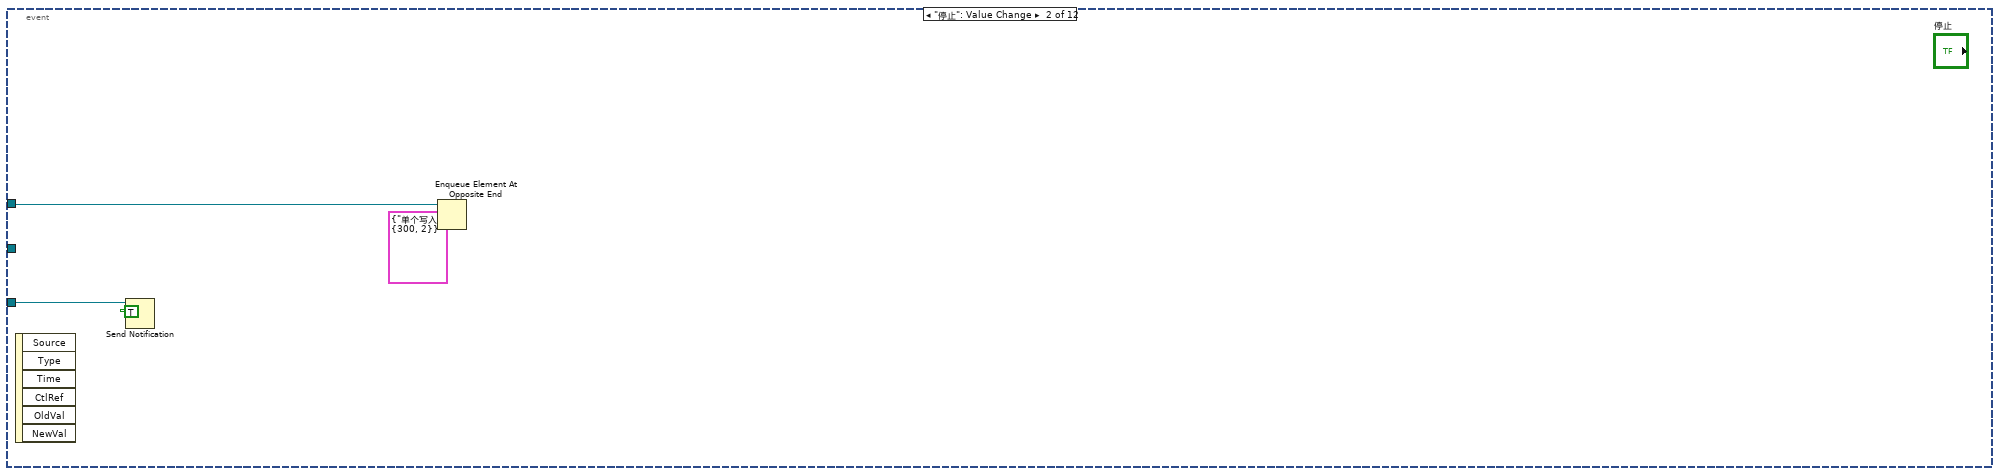
[diagram p19: hidden frame]
diagram:
  n1 = while {
    stop <- FALSE stop-if-true
    n2 = local read "R111"() -> (w35:u16)
    n3 = Wait (ms)(milliseconds to wait=u32 1000 ("等待时间（毫秒）")) -> ()  [unwired: 1 out]
    n4 = Not Equal To 0?(x=w35) -> (x != 0?=w34:bool)
    n5 = case shown="假" w34 {
      tunnel: [_ TRUE ("可见")] -> w26
      tunnel: ["二级进样切换阀_V6-G" ("布尔文本.文本") "过滤装置排液阀_V6" ("布尔文本.文本")] -> w32
      tunnel: ["过滤切换阀_V6-R" ("布尔文本.文本") "过滤三通阀1_V7-G" ("布尔文本.文本")] -> w31
      tunnel: ["空压机出气阀_V7" ("布尔文本.文本") "空压机出气阀_V10" ("布尔文本.文本")] -> w30
      tunnel: ["自来水出水阀_V8" ("布尔文本.文本") "自来水出水阀_V11" ("布尔文本.文本")] -> w29
      tunnel: ["采水泵1反冲洗阀_V9" ("布尔文本.文本") "采水泵1反冲洗阀_V12" ("布尔文本.文本")] -> w28
      tunnel: ["采水泵2反冲洗阀_V10" ("布尔文本.文本") "采水泵2反冲洗阀_V13" ("布尔文本.文本")] -> w27
      frame False {
      }
      frame True {
      }
    }
    n6 = property on="R103" class="DigNum (严格)"("Visible"=w26) -> ()  [unwired: 2 in, 2 out]
    n7 = property on="R104" class="DigNum (严格)"("Visible"=w26) -> ()  [unwired: 2 in, 2 out]
    n8 = property on="R110" class="DigNum (严格)"("Visible"=w26) -> ()  [unwired: 2 in, 2 out]
    n9 = property on="R44" class="DigNum (严格)"("Visible"=w26) -> ()  [unwired: 2 in, 2 out]
    n10 = property on="R107" class="DigNum (严格)"("Visible"=w26) -> ()  [unwired: 2 in, 2 out]
    n11 = property on="V14" class="Bool (严格)"("Visible"=w26) -> ()  [unwired: 2 in, 2 out]
    n12 = property on="V9" class="Bool (严格)"("Visible"=w26) -> ()  [unwired: 2 in, 2 out]
    n13 = property on="数值 11" class="DigNum (严格)"("Visible"=w26) -> ()  [unwired: 2 in, 2 out]
    n14 = property on="V7-R" class="Bool (严格)"("Visible"=w26) -> ()  [unwired: 2 in, 2 out]
    n15 = property on="V8" class="Bool (严格)"("Visible"=w26) -> ()  [unwired: 2 in, 2 out]
    n16 = property on="数值 10" class="DigNum (严格)"("Visible"=w26) -> ()  [unwired: 2 in, 2 out]
    n17 = property on="数值 9" class="DigNum (严格)"("Visible"=w26) -> ()  [unwired: 2 in, 2 out]
    n18 = property on="V13" class="Bool (严格)"("BoolText.Text"=w27) -> ()  [unwired: 2 in, 2 out]
    n19 = property on="V12" class="Bool (严格)"("BoolText.Text"=w28) -> ()  [unwired: 2 in, 2 out]
    n20 = property on="V11" class="Bool (严格)"("BoolText.Text"=w29) -> ()  [unwired: 2 in, 2 out]
    n21 = property on="V10" class="Bool (严格)"("BoolText.Text"=w30) -> ()  [unwired: 2 in, 2 out]
    n22 = property on="V7-G" class="Bool (严格)"("BoolText.Text"=w31) -> ()  [unwired: 2 in, 2 out]
    n23 = property on="V6" class="Bool (严格)"("BoolText.Text"=w32) -> ()  [unwired: 2 in, 2 out]
  }
  n24 = flat-sequence {
    frame #0 {
      n25 = property on="窗格" class="Pane"("Origin"=T2 {"Horizontal"=0, "Vertical"=0} ("原点")) -> ()  [unwired: 2 in, 2 out]
    }
  }
  n26 = Obtain Queue(name (unnamed)="采配水" ("名称（未命名）"), element data type=cluster{"命令":string, "数据":variant} {"命令"="", "数据"=variant}) -> (queue out=w4:refnum<queue>)  [unwired: 3 in, 2 out]
  n27 = Obtain Queue(name (unnamed)="采配水" ("名称（未命名）"), element data type=cluster{"命令":string, "数据":variant} {"命令"="", "数据"=variant}) -> (queue out=w15:refnum<queue>, error out=w14:errorcluster)  [unwired: 3 in, 1 out]
  n28 = Obtain Notifier(name (unnamed)="采配水Process" ("名称（未命名）"), notification data type=FALSE) -> (notifier out=w18:refnum<notifier>)  [unwired: 2 in, 2 out]
  n29 = while {
    tunnel: w4 -> [w55]
    stop <- FALSE stop-if-true
    # "看门狗定时喂狗"
    n30 = Wait (ms)(milliseconds to wait=u32 5000 ("等待时间（毫秒）")) -> ()  [unwired: 1 out]
    n31 = Bundle By Name(cluster=T3 {"命令"="单个写入", "数据"={"starting address"=0, "holding register value"=0}} ("元素"), "数据.starting address"=u16 56, "数据.holding register value"=u16 0) -> (w56:T3)
    n32 = Enqueue Element At Opposite End(queue=w55, element=w56) -> ()  [unwired: 2 in, 3 out]
  }
  n33 = Obtain Queue(name (unnamed)="采配水" ("名称（未命名）"), element data type=cluster{"命令":string, "数据":variant} {"命令"="", "数据"=variant}) -> (queue out=w22:refnum<queue>, error out=w23:errorcluster)  [unwired: 3 in, 1 out]
  n34 = Obtain Queue(name (unnamed)="taskprocess" ("名称（未命名）"), element data type=T1 {"测试模式"=enum."水样测试", "参数启用"={"氨氮"=FALSE, "总磷"=FALSE, "总氮"=FALSE, "多参数"=FALSE, "CODMn"=FALSE, "CODcr"=FALSE, "超标留样"=FALSE}} ("参数")) -> (queue out=w2:refnum<queue>)  [unwired: 3 in, 2 out]
  n35 = while {
    tunnel: w22 -> [w60]
    tunnel: w23 -> [_]
    tunnel: w18 -> [w59]
    tunnel: w2 -> [w58]
    stop <- FALSE stop-if-true
    n36 = event shown="[2] \"启动\": 值改变" {
      selector: _ -> [_ _ _ _ _ _ _ _ _ _ _ _]
      dyn-events: _ -> [_ _ _ _ _ _ _ _ _ _ _ _]
      timeout: _ -> [_ _ _ _ _ _ _ _ _ _ _ _]
      tunnel: w60 -> [_ w64 _ w86 w105 w114 w119 _ _ _ w153 w157]
      tunnel: w59 -> [_ w63 w68 _ _ _ _ _ _ _ _ _]
      tunnel: w58 -> [_ _ w66 _ _ _ _ _ _ _ _ _]
      event Timeout {
        n37 = event-data() -> ()  [unwired: 1 in, 3 out]
      }
      event "停止": Value Change {
        n38 = event-data() -> ()  [unwired: 1 in, 6 out]
        n39 = Send Notification(notification=TRUE ("通知"), notifier=w63) -> ()  [unwired: 1 in, 2 out]
        n40 = Enqueue Element At Opposite End(queue=w64, element=T4 {"命令"="单个写入", {"starting address"=300, "holding register value"=2}} ("元素")) -> ()  [unwired: 2 in, 3 out]
      }
      event "启动": Value Change {
        n41 = event-data() -> ()  [unwired: 1 in, 6 out]
        n42 = flat-sequence {
          tunnel: w68 -> [w70]
          tunnel: [w69] -> w67
          tunnel: w66 -> [w69]
          tunnel: w67 -> [w71]
          frame #0 {
            n43 = Cancel Notification(0:w70) -> ()  [unwired: 1 in, 3 out]
          }
          frame #1 {
            n44 = call "手动启动选择对话框.vi"() -> ("确定"=w73:bool, "输出簇"=w72:T7)  [unwired: 10 in]
            n45 = case shown="真" w73 {
              tunnel: w72 -> [_ w75]
              tunnel: w71 -> [_ w74]
              frame False {
              }
              frame True {
                n46 = global read "采配水全局变量.vi" "流程运行中"() -> (w76:bool)
                n47 = case shown="假" w76 {
                  tunnel: w75 -> [w79 _]
                  tunnel: w74 -> [w81 _]
                  frame False {
                    n48 = Unbundle By Name(w79) -> ("参数启用"=w78:T8)
                    n49 = Bundle("测试模式"=enum16{"水样测试", "平行样测试", "集成干预测试", "加标回收"}."水样测试", "参数启用"=w78) -> (w77:T9)  [unwired: 1 in]
                    n50 = Enqueue Element(queue=w81, element=w77) -> ()  [unwired: 2 in, 3 out]
                  }
                  frame True {
                    n51 = One Button Dialog(message="流程已启动，无需重复启动！" ("消息")) -> ()  [unwired: 1 in, 1 out]
                  }
                }
              }
            }
          }
        }
      }
      event "单步启动": Value Change {
        n52 = event-data() -> ()  [unwired: 1 in, 6 out]
        n53 = call "单步启动对话框.vi"() -> ("单步启动步骤输出"=w83:u16)  [unwired: 11 in]
        n54 = Bundle By Name(cluster=T3 {"命令"="单个写入", "数据"={"starting address"=301, "holding register value"=0}} ("元素"), "数据.holding register value"=w83) -> (w84:T3)
        n55 = Enqueue Element At Opposite End(queue=w86, element=w84) -> ()  [unwired: 2 in, 3 out]
      }
      event "R101", "R102", "R103", "R104", "R105", "R106", "R107", "R108", "R109", "R100", "R110", "R111", "R112", "R113": Value Change {
        n56 = event-data() -> ()  [unwired: 1 in, 6 out]
        n57 = local read "R101"() -> (w101:i16)
        n58 = local read "R102"() -> (w100:i16)
        n59 = local read "R103"() -> (w99:i16)
        n60 = local read "R104"() -> (w98:i16)
        n61 = local read "R105"() -> (w97:i16)
        n62 = local read "R106"() -> (w96:i16)
        n63 = local read "R107"() -> (w95:i16)
        n64 = local read "R108"() -> (w94:i16)
        n65 = local read "R109"() -> (w92:i16)
        n66 = local read "R110"() -> (w91:i16)
        n67 = local read "R112"() -> (w88:i16)
        n68 = Build Array("R100", w101, w100, w99, w98, w97, w96, w95, w94, w92, w91, "R111", w88, "R113") -> (w90:u16[])
        n69 = Bundle By Name(cluster=T5 {"命令"="多个写入", "数据"={"starting address"=0, "holding register values"=[]}} ("元素"), "数据.starting address"=u16 100, "数据.holding register values"=w90) -> (w102:T5)
        n70 = Enqueue Element At Opposite End(queue=w105, element=w102) -> ()  [unwired: 2 in, 3 out]
      }
      event "R116", "R117", "R118", "R120", "R121", "R122": Value Change {
        n71 = event-data() -> ()  [unwired: 1 in, 6 out]
        n72 = local read "R116"() -> (w112:i16)
        n73 = local read "R117"() -> (w111:i16)
        n74 = local read "R120"() -> (w109:i16)
        n75 = local read "R121"() -> (w108:i16)
        n76 = local read "R122"() -> (w107:i16)
        n77 = Build Array(w112, w111, "R118", i16 0 ("R116"), w109, w108, w107) -> (w113:u16[])
        n78 = Bundle By Name(cluster=T5 {"命令"="多个写入", "数据"={"starting address"=0, "holding register values"=[]}} ("元素"), "数据.starting address"=u16 116, "数据.holding register values"=w113) -> (w115:T5)
        n79 = Enqueue Element At Opposite End(queue=w114, element=w115) -> ()  [unwired: 2 in, 3 out]
      }
      event "R124": Value Change {
        n80 = event-data() -> ("NewVal"=w118:i16)  [unwired: 1 in, 5 out]
        n81 = Build Array(w118) -> (w120:i16[])
        n82 = Bundle By Name(cluster=T5 {"命令"="多个写入", "数据"={"starting address"=0, "holding register values"=[]}} ("元素"), "数据.starting address"=u16 124, "数据.holding register values"=w120) -> (w121:T5)
        n83 = Enqueue Element At Opposite End(queue=w119, element=w121) -> ()  [unwired: 2 in, 3 out]
      }
      event "R101", "R102", "R103", "R104", "R105", "R106", "R107", "R108", "R109", "R117", "R110", "R116", "R112", "R120", "R121", "R122", "R124": Mouse Down {
        n84 = event-data() -> ("CtlRef"=w127:refnum<vi>)  [unwired: 1 in, 7 out]
        n85 = property class="DigNum (严格)"(reference=w127) -> (reference out=w125:refnum<vi>, "Value"=w126:i16)  [unwired: 1 in, 1 out]
        n86 = call "数字键盘.vi"("OldNumber"=w126) -> ("NewNumber"=w124:sgl)
        n87 = property class="DigNum (严格)"(reference=w125, "Val(Sgnl)"=w124) -> ()  [unwired: 1 in, 2 out]
      }
      event "参数设置": Value Change {
        n88 = event-data() -> ()  [unwired: 1 in, 6 out]
        n89 = property on="窗格" class="Pane"("Origin"=T2 {"Horizontal"=0, "Vertical"=628} ("原点")) -> ()  [unwired: 2 in, 2 out]
      }
      event "返回": Value Change {
        n90 = event-data() -> ()  [unwired: 1 in, 6 out]
        n91 = property on="窗格" class="Pane"("Origin"=T2 {"Horizontal"=0, "Vertical"=0} ("原点")) -> ()  [unwired: 2 in, 2 out]
      }
      event "M1", "M2", "V2", "V3", "V4", "V5", "V6", "V7-G", "V7-R", "V8", "V9", "V10", "V11", "V1-G", "V1-R", "V12", "V13", "M4", "M3", "V14": Value Change {
        n92 = event-data() -> ()  [unwired: 1 in, 6 out]
        n93 = Build Array("V1-G", "V1-R", "V2", "V3", "V4", "V5", "V6", "V7-G", "V7-R", "V8", "V9", "V10", "V11", "V12", "V13", "M1", "M2", "M3", "M4", "V14") -> (w146:bool[])
        n94 = Bundle By Name(cluster=T6 {"命令"="线圈写入", "data"={"starting address"=2400, "coil values"=[]}} ("元素"), "data.coil values"=w146) -> (w147:T6)
        n95 = Enqueue Element(queue=w153, element=w147) -> ()  [unwired: 2 in, 3 out]
      }
      event "更新程序": Value Change {
        n96 = event-data() -> ("NewVal"=w154:bool)  [unwired: 1 in, 5 out]
        n97 = case shown="真" w154 {
          tunnel: [cluster{"命令":string, "数据":variant} {"命令"="init", "数据"=variant} ("元素") w161] -> w156
          frame False {
          }
          frame True {
            n98 = Two Button Dialog(message="警告，非专业人士请勿进行此操作！！！\n请确认是否释放串口？" ("消息")) -> (T button?=w160:bool)  [unwired: 2 in]
            n99 = case shown="真" w160 {
              tunnel: [_ cluster{"命令":string, "数据":variant} {"命令"="shutdown", "数据"=variant} ("元素")] -> w161
              frame False {
                n100 = local write "更新程序"(FALSE ("释放串口")) -> ()
              }
              frame True {
              }
            }
          }
        }
        n101 = Flush Queue(queue=w157) -> (queue out=w155:refnum<queue>)  [unwired: 1 in, 2 out]
        n102 = Enqueue Element(queue=w155, element=w156) -> ()  [unwired: 2 in, 3 out]
      }
    }
  }
  n103 = Enqueue Element(queue=w15, element=cluster{"命令":string, "数据":variant} {"命令"="init", "数据"=variant} ("元素"), error in (no error)=w14) -> (queue out=w10:refnum<queue>, error out=w12:errorcluster)  [unwired: 1 in, 1 out]
  n104 = while {
    tunnel: w22 -> [w180]
    stop <- FALSE stop-if-true
    n105 = global read "采配水全局变量.vi" "状态"() -> (w178:T10)
    n106 = Wait (ms)(milliseconds to wait=u32 1000 ("等待时间（毫秒）")) -> ()  [unwired: 1 out]
    n107 = global read "采配水全局变量.vi" "报警簇"() -> (w174:bool[])
    n108 = Unbundle By Name(w178) -> ("R0"=w168:i16, "R1"=→"R1":i16, "R2"=→"R2":i16, "R54"=→"清洗次数":i16, "R47"=→"当前启动泵号":i16, "R44"=→"R44":i16)  [unwired: 1 out]
    "多列列表框" <- w168
    n109 = Enqueue Element(queue=w180, element=cluster{"命令":string, "数据":variant} {"命令"="读状态", "数据"=variant} ("元素")) -> (queue out=w170:refnum<queue>)  [unwired: 2 in, 2 out]
    n110 = call "报警信息.vi"("报警簇"=w174) -> ("采配水报警信息"=w167:string)  [unwired: 9 in, 1 out]
    n111 = case shown="默认" w167 {
      selector: w167 -> [w182 _]
      tunnel: [w182 w183] -> w173
      frame Default {
      }
      frame "" {
        n112 = global read "采配水全局变量.vi" "运行状态显示"() -> (w183:string)
      }
    }
    "集成报警信息" <- w173
    n113 = Enqueue Element(queue=w170, element=cluster{"命令":string, "数据":variant} {"命令"="读参数", "数据"=variant} ("元素")) -> ()  [unwired: 2 in, 3 out]
    n114 = feedback-in #1(w168) -> ()
    n115 = feedback #1(w168) -> (w169:i16)
    n116 = Not Equal?(x=w169, y=w168) -> (x != y?=w175:bool)
    n117 = case shown="真" w175 {
      tunnel: w168 -> [_ w186]
      frame False {
      }
      frame True {
        n118 = property on="多列列表框" class="MCListbox (严格)"() -> ("ItemNames"=w187:string[][])  [unwired: 2 in, 2 out]
        n119 = Index Array(array=w187, index (row)=w186) -> (element=w185:string[])  [unwired: 1 in]
        n120 = Index Array(array=w185) -> (element=w184:string)  [unwired: 1 in]
        n121 = case shown="默认" w184 {
          selector: w184 -> [_ w188]
          frame "待机" {
          }
          frame Default {
            n122 = case shown="默认" w188 {
              selector: w188 -> [w194 _ _]
              tunnel: [w194 "-->>启动" "-->>结束"] -> w190
              frame Default {
              }
              frame "初始化" {
              }
              frame "结束" {
              }
            }
            n123 = Get Date/Time In Seconds() -> (seconds since 1Jan1904=w193:timestamp)
            n124 = Bundle("seconds since 1Jan1904"=w193, "table输入"="采配水", w190, "table输入"="") -> (w189:T11)  [unwired: 1 in]
            n125 = call "操作日志数据插入.vi"("data"=w189) -> ()  [unwired: 9 in, 1 out]
          }
        }
      }
    }
  }
  n126 = property on="多列列表框" class="MCListbox (严格)"("ItemNames"=string[][] [["待机"], ["初始化"], ["水样润洗"], ["一级水样池进样"], ["二级水样池进样"], ["一级补充水样/沉淀"], ["配水"], ["反冲洗"], ["采样池储水"], ["结束"]] ("项名")) -> ()  [unwired: 2 in, 2 out]
  n127 = while {
    tunnel: w10 -> [w201]
    tunnel: w12 -> [w200]
    shift-right: [w204] -> w7
    shift-left: refnum<class "MB_Master.lvclass"> refnum ("MB session in") -> [w203]
    tunnel: errorcluster {"status"=FALSE, "code"=0, "source"=""} ("error out") -> [w202]
    tunnel: [w199] -> w8
    stop <- FALSE stop-if-true
    n128 = case shown="无错误" w202 {
      selector: w202 -> [w210 w406]
      tunnel: [w213 w405] -> w204
      tunnel: w203 -> [w212 w407]
      tunnel: [w211 w403] -> w199
      tunnel: w201 -> [w207 w402]
      tunnel: w200 -> [w206 _]
      tunnel: [w208 _] -> _
      frame No Error {
        n129 = Dequeue Element(queue=w207, error in (no error)=w206) -> (element=w205:cluster{"命令":string, "数据":variant})  [unwired: 1 in, 3 out]
        n130 = Unbundle By Name(w205) -> ("命令"=w209:string)
        n131 = case shown="\"读状态\"" w209 {
          tunnel: [w215 w216 w238 w356 w368 w378 w388 w399] -> w213
          tunnel: w212 -> [w215 w230 w322 w361 w371 w381 w391 w399]
          tunnel: [w214 w229 w239 w355 w369 w379 w389 w392] -> w211
          tunnel: w210 -> [w214 w232 w325 w360 w370 w380 w390 w395]
          tunnel: [_ _ _ _ _ _ _ TRUE] -> w208
          tunnel: w205 -> [_ _ _ _ w367 w377 w387 _]
          frame "idle", Default {
          }
          frame "init" {
            w220 = refnum<visa-resource-name> "COM3" ("VISA resource name")
            n132 = call-dynamic "Close Session.vi"("error in (no error)"=w232, "MB session in"=w230) -> ("error out"=w231:errorcluster)  [unwired: 9 in]
            n133 = call <vilib>:"Clear Errors.vi"("error in (no error)"=w231) -> ("error out"=w218:errorcluster)  [unwired: 5 in, 1 out]
            n134 = call-poly "VISA Configure Serial Port"("VISA resource name"=w220, "baud rate (9600)"=u32 115200, "error in (no error)"=w218) -> ("VISA resource name out"=w225:refnum<visa-resource-name>, "error out"=w224:errorcluster)  [unwired: 11 in]
            n135 = VISA Write(VISA resource name=w225, write buffer="\u0002004701R04047560A5B\u0003" ("写入缓冲区"), error in (no error)=w224) -> (VISA resource name out=w223:refnum<visa-resource-name>, error out=w222:errorcluster)  [unwired: 1 out]
            n136 = VISA Close(VISA resource name=w223, error in (no error)=w222) -> (error out=w217:errorcluster)
            n137 = call <vilib>:"Open Serial Session.vi"("Mode (RTU)"=enum16{"RTU", "ASCII"}."RTU", "Error in"=w217, "Slave ID"=u8 10, "Serial Config"=T12 {"baud rate (bps)"=115200, "stop bits"=10, "parity"=0, "flow control"=0, "timeout"=500, "retries"=1}, "VISA Resource"=w220) -> ("Error out"=w229:errorcluster, "MB_Serial session"=w216:refnum<class "MB_Master_Serial.lvclass">)  [unwired: 5 in]
            n138 = Unbundle By Name(w229) -> ("status"=w233:bool)
            n139 = global write "采配水全局变量.vi" "MB session in"(w216) -> ()
            n140 = call "对话框信息"("Enable"=w233) -> ()  [unwired: 9 in, 2 out]
          }
          frame "读状态" {
            # "压力传感器\n4-20  mA \n \n0-8191\n\n0-1MPA"
            n141 = call <vilib>:"Read Holding Registers.vi"("error in (no error)"=w325, "quantity"=u16 80 ("number of holding registers"), "starting address"=u16 0, "MB session in"=w322) -> ("error out"=w320:errorcluster, "Registers"=w264:u16[], "MB session out"=w321:refnum<class "MB_Master.lvclass">)  [unwired: 5 in]
            "Registers" <- w264
            n142 = Array Subset(array=w264, index=48 ("索引")) -> (w290:u16[])  [unwired: 1 in]
            n143 = Index Array(array=w264, index #1=13 ("索引")) -> (element #1=→"数值":u16, element #2=→"数值 2":u16, element #3=→"数值 3":u16, element #4=→"数值 4":u16, element #5=→"数值 5":u16, element #6=→"数值 6":u16, element #7=→"数值 7":u16, element #8=→"数值 8":u16, element #9=→"数值 9":u16, element #10=→"数值 10":u16, element #11=→"数值 11":u16, element #12=→"数值 12":u16, element #13=→"数值 13":u16, element #14=→"数值 14":u16, element #15=→"数值 15":u16, element #16=→"数值 16":u16, element #17=→"数值 17":u16, element #18=→"数值 18":u16, element #19=→"数值 19":u16)  [unwired: 18 in]
            n144 = call <vilib>:"Read Holding Registers.vi"("error in (no error)"=w320, "quantity"=u16 6 ("number of holding registers"), "starting address"=u16 3840, "MB session in"=w321) -> ("error out"=w316:errorcluster, "Registers"=w293:u16[], "MB session out"=w317:refnum<class "MB_Master.lvclass">)  [unwired: 5 in]
            n145 = Array To Cluster(array=w264) -> (cluster=w243:T16)
            n146 = global write "采配水全局变量.vi" "状态"(w243) -> ()
            n147 = To Word Integer(number=w293) -> (16bit integer=w292:i16[])
            n148 = Array To Cluster(array=w293) -> (cluster=w332:T17)
            n149 = global write "采配水全局变量.vi" "AD"(w332) -> ()
            n150 = call <vilib>:"Read Coils.vi"("error in (no error)"=w316, "quantity"=u16 32 ("number of coils"), "starting address"=u16 0, "MB session in"=w317) -> ("error out"=w312:errorcluster, "Coils"=w297:bool[], "MB session out"=w313:refnum<class "MB_Master.lvclass">)  [unwired: 5 in]
            n151 = call "FATEK_HexToString.vi"("数组"=w290) -> ("STRING"=w289:string[])  [unwired: 10 in]
            n152 = global write "采配水全局变量.vi" "输出状态"(w297) -> ()
            n153 = Index Array(array=w289) -> (element=→"采配水版本号":string)  [unwired: 1 in]
            n154 = Index Array(array=w297, index #20=31 ("索引")) -> (element #1=w271:bool, element #2=w287:bool, element #3=w286:bool, element #4=w285:bool, element #5=w284:bool, element #6=w283:bool, element #7=w282:bool, element #8=w278:bool, element #9=w277:bool, element #10=w276:bool, element #11=w275:bool, element #12=w274:bool, element #13=w273:bool, element #14=w270:bool, element #15=w269:bool, element #16=w268:bool, element #17=w267:bool, element #18=w266:bool, element #19=w265:bool, element #20=w241:bool)  [unwired: 19 in]
            n155 = formula code="float AD0,AD1,AD2,AD3,AD4,AD5,AD6;\n\nAD0 = IN[0]*140/6553-75;\nAD1 = IN[1]/65.53-25;\nAD2 = (IN[2]/65.53-25)/100;\nAD3 = IN[3]*30/8191;\nAD4 = IN[4]*30/8191;\nAD5 = IN[5]*30/8191;"("IN"=w292) -> ("AD0"=w330:dbl, "AD1"=w329:dbl, "AD2"=w272:dbl, "AD3"=w328:dbl, "AD4"=w327:dbl, "AD5"=w326:dbl)
            "压力传感器" <- w272
            n156 = call <vilib>:"Read Coils.vi"("error in (no error)"=w312, "quantity"=u16 16 ("number of coils"), "starting address"=u16 1000, "MB session in"=w313) -> ("error out"=w308:errorcluster, "Coils"=w304:bool[], "MB session out"=w309:refnum<class "MB_Master.lvclass">)  [unwired: 5 in]
            n157 = local write "V1-G"(w271) -> ()
            n158 = local write "V1-R"(w287) -> ()
            n159 = local write "V2"(w286) -> ()
            n160 = local write "V3"(w285) -> ()
            n161 = local write "V4"(w284) -> ()
            n162 = local write "V5"(w283) -> ()
            n163 = local write "V6"(w282) -> ()
            n164 = local write "V7-G"(w278) -> ()
            n165 = local write "V7-R"(w277) -> ()
            n166 = local write "V8"(w276) -> ()
            n167 = local write "V9"(w275) -> ()
            n168 = local write "V10"(w274) -> ()
            n169 = local write "V11"(w273) -> ()
            n170 = local write "V12"(w270) -> ()
            n171 = local write "V13"(w269) -> ()
            n172 = local write "M1"(w268) -> ()
            n173 = local write "M2"(w267) -> ()
            n174 = local write "M3"(w266) -> ()
            n175 = local write "M4"(w265) -> ()
            n176 = local write "V14"(w241) -> ()
            n177 = global write "采配水全局变量.vi" "输入状态"(w304) -> ()
            n178 = Bundle(w330, w329, w272, w328, w327, w326) -> (w331:cluster{dbl, dbl, dbl, dbl, dbl, dbl})  [unwired: 1 in]
            n179 = Index Array(array=w304) -> (element #1=→"X0":bool, element #2=→"X1":bool, element #3=→"X2":bool, element #4=→"X3":bool, element #5=→"X4":bool, element #6=→"X5":bool, element #7=→"X6":bool, element #8=→"X7":bool, element #9=→"X8":bool, element #10=→"X9":bool, element #11=→"X10":bool, element #12=→"X11":bool)  [unwired: 12 in]
            n180 = global write "采配水全局变量.vi" "转换值"(w331) -> ()
            n181 = call <vilib>:"Read Coils.vi"("error in (no error)"=w308, "quantity"=u16 16 ("number of coils"), "starting address"=u16 2500, "MB session in"=w309) -> ("error out"=w239:errorcluster, "Coils"=w305:bool[], "MB session out"=w240:refnum<class "MB_Master.lvclass">)  [unwired: 5 in]
            n182 = global write "采配水全局变量.vi" "报警簇"(w305) -> ()
            n183 = call <vilib>:"Read Coils.vi"("quantity"=u16 1, "starting address"=u16 2800, "MB session in"=w240) -> ("Coils"=w235:bool[], "MB session out"=w238:refnum<class "MB_Master.lvclass">)  [unwired: 6 in, 1 out]
            n184 = Index Array(array=w235) -> (element=w234:bool)  [unwired: 1 in]
            n185 = global write "采配水全局变量.vi" "看门狗启用"(w234) -> ()
          }
          frame "读参数" {
            n186 = call <vilib>:"Read Holding Registers.vi"("error in (no error)"=w360, "quantity"=u16 25 ("number of holding registers"), "starting address"=u16 100, "MB session in"=w361) -> ("error out"=w355:errorcluster, "Registers"=w357:u16[], "MB session out"=w356:refnum<class "MB_Master.lvclass">)  [unwired: 5 in]
            n187 = Array To Cluster(array=w357) -> (cluster=w345:T18)
            n188 = global write "采配水全局变量.vi" "参数设置"(w345) -> ()
            n189 = Unbundle(w345) -> ("Registers[0]"=w344:u16, "Registers[1]"=→"R101":u16, "Registers[2]"=→"R102":u16, "Registers[3]"=→"R103":u16, "Registers[4]"=→"R104":u16, "Registers[5]"=→"R105":u16, "Registers[6]"=→"R106":u16, "Registers[7]"=→"R107":u16, "Registers[8]"=→"R108":u16, "Registers[9]"=→"R109":u16, "Registers[10]"=→"R110":u16, "Registers[11]"=w341:u16, "Registers[12]"=→"R112":u16, "Registers[13]"=w339:u16, "Registers[16]"=→"R116":u16, "Registers[17]"=→"R117":u16, "Registers[18]"=w337:u16, "Registers[20]"=→"R120":u16, "Registers[21]"=→"R121":u16, "Registers[22]"=→"R122":u16, "Registers[24]"=→"R124":u16)  [unwired: 13 out]
            n190 = local write "R100"(w344) -> ()
            n191 = local write "R111"(w341) -> ()
            n192 = local write "R113"(w339) -> ()
            n193 = local write "R118"(w337) -> ()
          }
          frame "多个写入" {
            n194 = Unbundle By Name(w367) -> ("数据"=w366:variant)
            n195 = Variant To Data(type=T13 {"starting address"=0, "holding register values"=[]}, Variant=w366) -> (data=w364:T13)  [unwired: 1 in, 1 out]
            n196 = Unbundle By Name(w364) -> ("starting address"=w363:u16, "holding register values"=w362:u16[])
            n197 = call <vilib>:"Write Multiple Registers.vi"("error in (no error)"=w370, "values"=w362, "starting address"=w363, "MB session in"=w371) -> ("error out"=w369:errorcluster, "MB session out"=w368:refnum<class "MB_Master.lvclass">)  [unwired: 6 in]
          }
          frame "单个写入" {
            n198 = Unbundle By Name(w377) -> ("数据"=w376:variant)
            n199 = Variant To Data(type=T14 {"starting address"=0, "holding register value"=0}, Variant=w376) -> (data=w374:T14)  [unwired: 1 in, 1 out]
            n200 = Unbundle By Name(w374) -> ("starting address"=w373:u16, "holding register value"=w372:u16)
            n201 = call <vilib>:"Write Single Register.vi"("error in (no error)"=w380, "value"=w372, "address"=w373, "MB session in"=w381) -> ("error out"=w379:errorcluster, "MB session out"=w378:refnum<class "MB_Master.lvclass">)  [unwired: 6 in]
          }
          frame "线圈写入" {
            n202 = Unbundle By Name(w387) -> ("数据"=w386:variant)
            n203 = Variant To Data(type=T15 {"starting address"=0, "coil values"=[]}, Variant=w386) -> (data=w384:T15)  [unwired: 1 in, 1 out]
            n204 = Unbundle By Name(w384) -> ("starting address"=w383:u16, "coil values"=w382:bool[])
            n205 = call <vilib>:"Write Multiple Coils.vi"("error in (no error)"=w390, "values"=w382, "starting address"=w383, "MB session in"=w391) -> ("error out"=w389:errorcluster, "MB session out"=w388:refnum<class "MB_Master.lvclass">)  [unwired: 6 in]
          }
          frame "shutdown" {
            n206 = call <vilib>:"Write Single Register.vi"("error in (no error)"=w395, "value"=u16 0, "address"=u16 4047, "MB session in"=w399) -> ("error out"=w394:errorcluster, "MB session out"=w398:refnum<class "MB_Master.lvclass">)  [unwired: 6 in]
            n207 = call-dynamic "Close Session.vi"("error in (no error)"=w394, "MB session in"=w398) -> ("error out"=w400:errorcluster)  [unwired: 9 in]
            n208 = call <vilib>:"Clear Errors.vi"("error in (no error)"=w400) -> ("error out"=w393:errorcluster)  [unwired: 5 in, 1 out]
            n209 = call "调用WinProladder.vi"("错误输入（无错误）"=w393) -> ("错误输出"=w392:errorcluster)  [unwired: 10 in]
          }
        }
      }
      frame Error {
        n210 = Unbundle By Name(w406) -> ("code"=w408:i32)
        n211 = case shown="-1073807343" w408 {
          tunnel: w407 -> [w410 w414]
          tunnel: w406 -> [w409 w416]
          tunnel: [w409 w415] -> w404
          tunnel: [w410 w414] -> w405
          tunnel: w402 -> [_ w413]
          frame Default {
          }
          frame -1073807343 {
            n212 = Flush Queue(queue=w413) -> (queue out=w412:refnum<queue>)  [unwired: 1 in, 2 out]
            n213 = call-dynamic "Close Session.vi"("error in (no error)"=w416, "MB session in"=w414) -> ("error out"=w415:errorcluster)  [unwired: 9 in]
            n214 = disable-structure shown="禁用" {
              disable-tunnel: w412 -> [w417 _]
              frame Disabled {
                n215 = Enqueue Element At Opposite End(queue=w417, element=cluster{"命令":string, "数据":variant} {"命令"="init", "数据"=variant} ("元素")) -> ()  [unwired: 2 in, 3 out]
              }
              frame Enabled {
              }
            }
            n216 = Wait (ms)(milliseconds to wait=u32 2000 ("等待时间（毫秒）")) -> ()  [unwired: 1 out]
          }
        }
        n217 = call <vilib>:"Clear Errors.vi"("error in (no error)"=w404) -> ("error out"=w403:errorcluster)  [unwired: 5 in, 1 out]
      }
    }
    n218 = Unbundle By Name(w199) -> ("status"=→"通讯故障":bool)
  }
  n219 = call-dynamic "Close Session.vi"("error in (no error)"=w8, "MB session in"=w7) -> ()  [unwired: 9 in, 1 out]
